vi "Grid_Monitor_V2backupblack.vi"(7 "Stop (In)":refnum<notifier>, 8 "Error (In)":errorcluster, 11 "SCADA AugState (In)":refnum<notifier>) -> (0 "Error (Out)":errorcluster, 3 "SCADA AugState (Out)":refnum<notifier>, 6 "Stop (Out)":refnum<notifier>)   [LabVIEW 2021]
uses:
  <vilib>/Utility/miscctls.llb/LVForegroundBackgroundColorsTypeDef.ctl
  SCADA/SCADA Augmented State.ctl
  Interval.ctl
  SCADA/SCADA Augmented State GUPTA.ctl
panel:
  out "V slider 11":T1(slide) caption="V-i" scale=230.0..240.0 scale format="%#_4g"
  out "V slider 25":dbl(slide) caption="V-i" max=-10.0 scale=720.0..750.0 scale format="%#_4g"
  out "V slider 24":dbl(slide) caption="V-i" max=-10.0 scale=720.0..750.0 scale format="%#_4g"
  out "V slider 23":dbl(slide) caption="V-i" max=-10.0 scale=720.0..750.0 scale format="%#_4g"
  out "V slider 22":dbl(slide) caption="V-i" max=-10.0 scale=720.0..750.0 scale format="%#_4g"
  out "V slider 21":dbl(slide) caption="V-i" max=-10.0 scale=720.0..750.0 scale format="%#_4g"
  out "V slider 20":dbl(slide) caption="V-i" max=-10.0 scale=720.0..750.0 scale format="%#_4g"
  out "V slider 19":dbl(slide) caption="V-i" max=-10.0 scale=720.0..750.0 scale format="%#_4g"
  out "V slider 18":dbl(slide) caption="V-i" max=-10.0 scale=720.0..750.0 scale format="%#_4g"
  out "V slider 17":T1(slide) caption="V-i" scale=230.0..240.0 scale format="%#_4g"
  out "V slider 16":T1(slide) caption="V-i" scale=230.0..240.0 scale format="%#_4g"
  out "V slider 15":T1(slide) caption="V-i" scale=230.0..240.0 scale format="%#_4g"
  out "V slider 14":T1(slide) caption="V-i" scale=230.0..240.0 scale format="%#_4g"
  out "V slider 13":T1(slide) caption="V-i" scale=230.0..240.0 scale format="%#_4g"
  out "V slider 12":T1(slide) caption="V-i" scale=230.0..240.0 scale format="%#_4g"
  out "V slider 10":T1(slide) caption="V-i" scale=230.0..240.0 scale format="%#_4g"
  out "V slider 9":T1(slide) caption="V-i" scale=230.0..240.0 scale format="%#_4g"
  out "V slider 8":T1(slide) caption="V-i" scale=230.0..240.0 scale format="%#_4g"
  out "V slider 7":T1(slide) caption="V-i" scale=230.0..240.0 scale format="%#_4g"
  out "V slider 6":T1(slide) caption="V-i" scale=230.0..240.0 scale format="%#_4g"
  out "V slider 4":T1(slide) caption="V-i" scale=230.0..240.0 scale format="%#_4g"
  out "V slider 3":T1(slide) caption="V-i" scale=230.0..240.0 scale format="%#_4g"
  out "V slider 1":T1(slide) caption="V-i" scale=230.0..240.0 scale format="%#_4g"
  out "V slider 0":T1(slide) caption="V-i" scale=230.0..240.0 scale format="%#_4g"
  out "size(s)":i32
  out "I slider 20":dbl(slide) min=-10.0 max=100.0 scale=0.0..100.0
  out "I slider 19":dbl(slide) min=-10.0 max=100.0 scale=0.0..100.0
  out "I slider 18":dbl(slide) min=-10.0 max=100.0 scale=0.0..100.0
  out "I slider 17":dbl(slide) min=-10.0 max=100.0 scale=0.0..100.0
  out "I slider 16":T1(slide) scale=0.0..44.0
  out "I slider 15":T1(slide) scale=0.0..44.0
  out "I slider 14":T1(slide) scale=0.0..44.0
  out "I slider 13":T1(slide) scale=0.0..44.0
  out "I slider 12":T1(slide) scale=0.0..108.0
  out "I slider 11":T1(slide) scale=0.0..82.0
  out "I slider 10":T1(slide) scale=0.0..82.0 scale format="%^#1.3g"
  out "I slider 9":T1(slide) scale=0.0..44.0
  out "I slider 8":T1(slide) scale=0.0..82.0 scale format="%^#1.3g"
  out "I slider 7":T1(slide) scale=0.0..207.0
  out "I slider 6":T1(slide) scale=0.0..135.0 scale format="%^#1.3g"
  out "I slider 5":T1(slide) scale=0.0..82.0
  out "I slider 4":T1(slide) scale=0.0..82.0
  out "I slider 3":T1(slide) scale=0.0..108.0
  out "I slider 2":T1(slide) scale=0.0..207.0 scale format="%^#1.3g"
  out "I slider 0":T1(slide) scale=0.0..207.0
  out "I slider 1":T1(slide) scale=0.0..44.0
  out "V slider 2":T1(slide) caption="V-i" scale=230.0..240.0 scale format="%#_4g"
  out "A":dbl caption="Numeric" format="%-^#10.3g"
  out "kW":dbl caption="Numeric" format="%#.3g"
  out "A":dbl caption="Numeric" format="%-^#10.3g"
  out "kW":dbl caption="Numeric" format="%#.3g"
  out "A":dbl caption="Numeric" format="%-^#10.3g"
  out "kW":dbl caption="Numeric" format="%#.3g"
  out "A":dbl caption="Numeric" format="%-^#10.3g"
  out "kW":dbl caption="Numeric" format="%#.3g"
  out "A":dbl caption="Numeric" format="%-^#10.3g"
  out "kW":dbl caption="Numeric" format="%#.3g"
  out "A":dbl caption="Numeric" format="%-^#10.3g"
  out "kW":dbl caption="Numeric" format="%#.3g"
  out "A":dbl caption="Numeric" format="%-^#10.3g"
  out "kW":dbl caption="Numeric" format="%#.3g"
  out "A":dbl caption="Numeric" format="%-^#10.3g"
  out "kW":dbl caption="Numeric" format="%#.3g"
  out "A":dbl[unit] caption="Numeric" format="%-^#10.3g"
  out "?VkVAr":dbl caption="Numeric" format="%.3g"
  out "kW":dbl caption="Numeric" format="%#.3g"
  out "A":dbl[unit] caption="Numeric" format="%-^#10.3g"
  out "?VkVAr":dbl caption="Numeric" format="%.3g"
  out "kW":dbl caption="Numeric" format="%#.3g"
  out "A":dbl[unit] caption="Numeric" format="%-^#10.3g"
  out "?VkVAr":dbl caption="Numeric" format="%.3g"
  out "kW":dbl caption="Numeric" format="%#.3g"
  out "A":dbl[unit] caption="Numeric" format="%-^#10.3g"
  out "?VkVAr":dbl caption="Numeric" format="%.3g"
  out "kW":dbl caption="Numeric" format="%#.3g"
  out "A":dbl[unit] caption="Numeric" format="%-^#10.3g"
  out "?VkVAr":dbl caption="Numeric" format="%.3g"
  out "kW":dbl caption="Numeric" format="%#.3g"
  out "A":dbl[unit] caption="Numeric" format="%-^#10.3g"
  out "?VkVAr":dbl caption="Numeric" format="%.3g"
  out "kW":dbl caption="Numeric" format="%#.3g"
  out "A":dbl[unit] caption="Numeric" format="%-^#10.3g"
  out "?VkVAr":dbl caption="Numeric" format="%.3g"
  out "kW":dbl caption="Numeric" format="%#.3g"
  out "A":dbl[unit] caption="Numeric" format="%-^#10.3g"
  out "?VkVAr":dbl caption="Numeric" format="%.3g"
  out "kW":dbl caption="Numeric" format="%#.3g"
  out "A":dbl[unit] caption="Numeric" format="%-^#10.3g"
  out "?VkVAr":dbl caption="Numeric" format="%.3g"
  out "kW":dbl caption="Numeric" format="%#.3g"
  out "A":dbl[unit] caption="Numeric" format="%-^#10.3g"
  out "?VkVAr":dbl caption="Numeric" format="%.3g"
  out "kW":dbl caption="Numeric" format="%#.3g"
  out "A2":dbl[unit] caption="Numeric" format="%-^#10.3g"
  out "?VkVAr":dbl caption="Numeric" format="%.3g"
  out "kW":dbl caption="Numeric" format="%#.3g"
  in  "Stop?":bool
  out "Connected?":bool
  out "AugState (Out)":refnum<notifier>
  in  "AugState (In)":refnum<notifier>
  # "B03"
  # "B01"
  # "B02"
  # "B05"
  # "B07"
  # "B14"
  # "B04"
  # "B06"
  # "B18"
  # "B22"
  # "B26"
  # "B08"
  # "B15"
  # "B19"
  # "B23"
  # "B09"
  # "B11"
  # "B10"
  # "B17"
  # "B21"
  # "B25"
  # "B13"
  # "B12"
  # "B16"
  # "B20"
  # "B24"
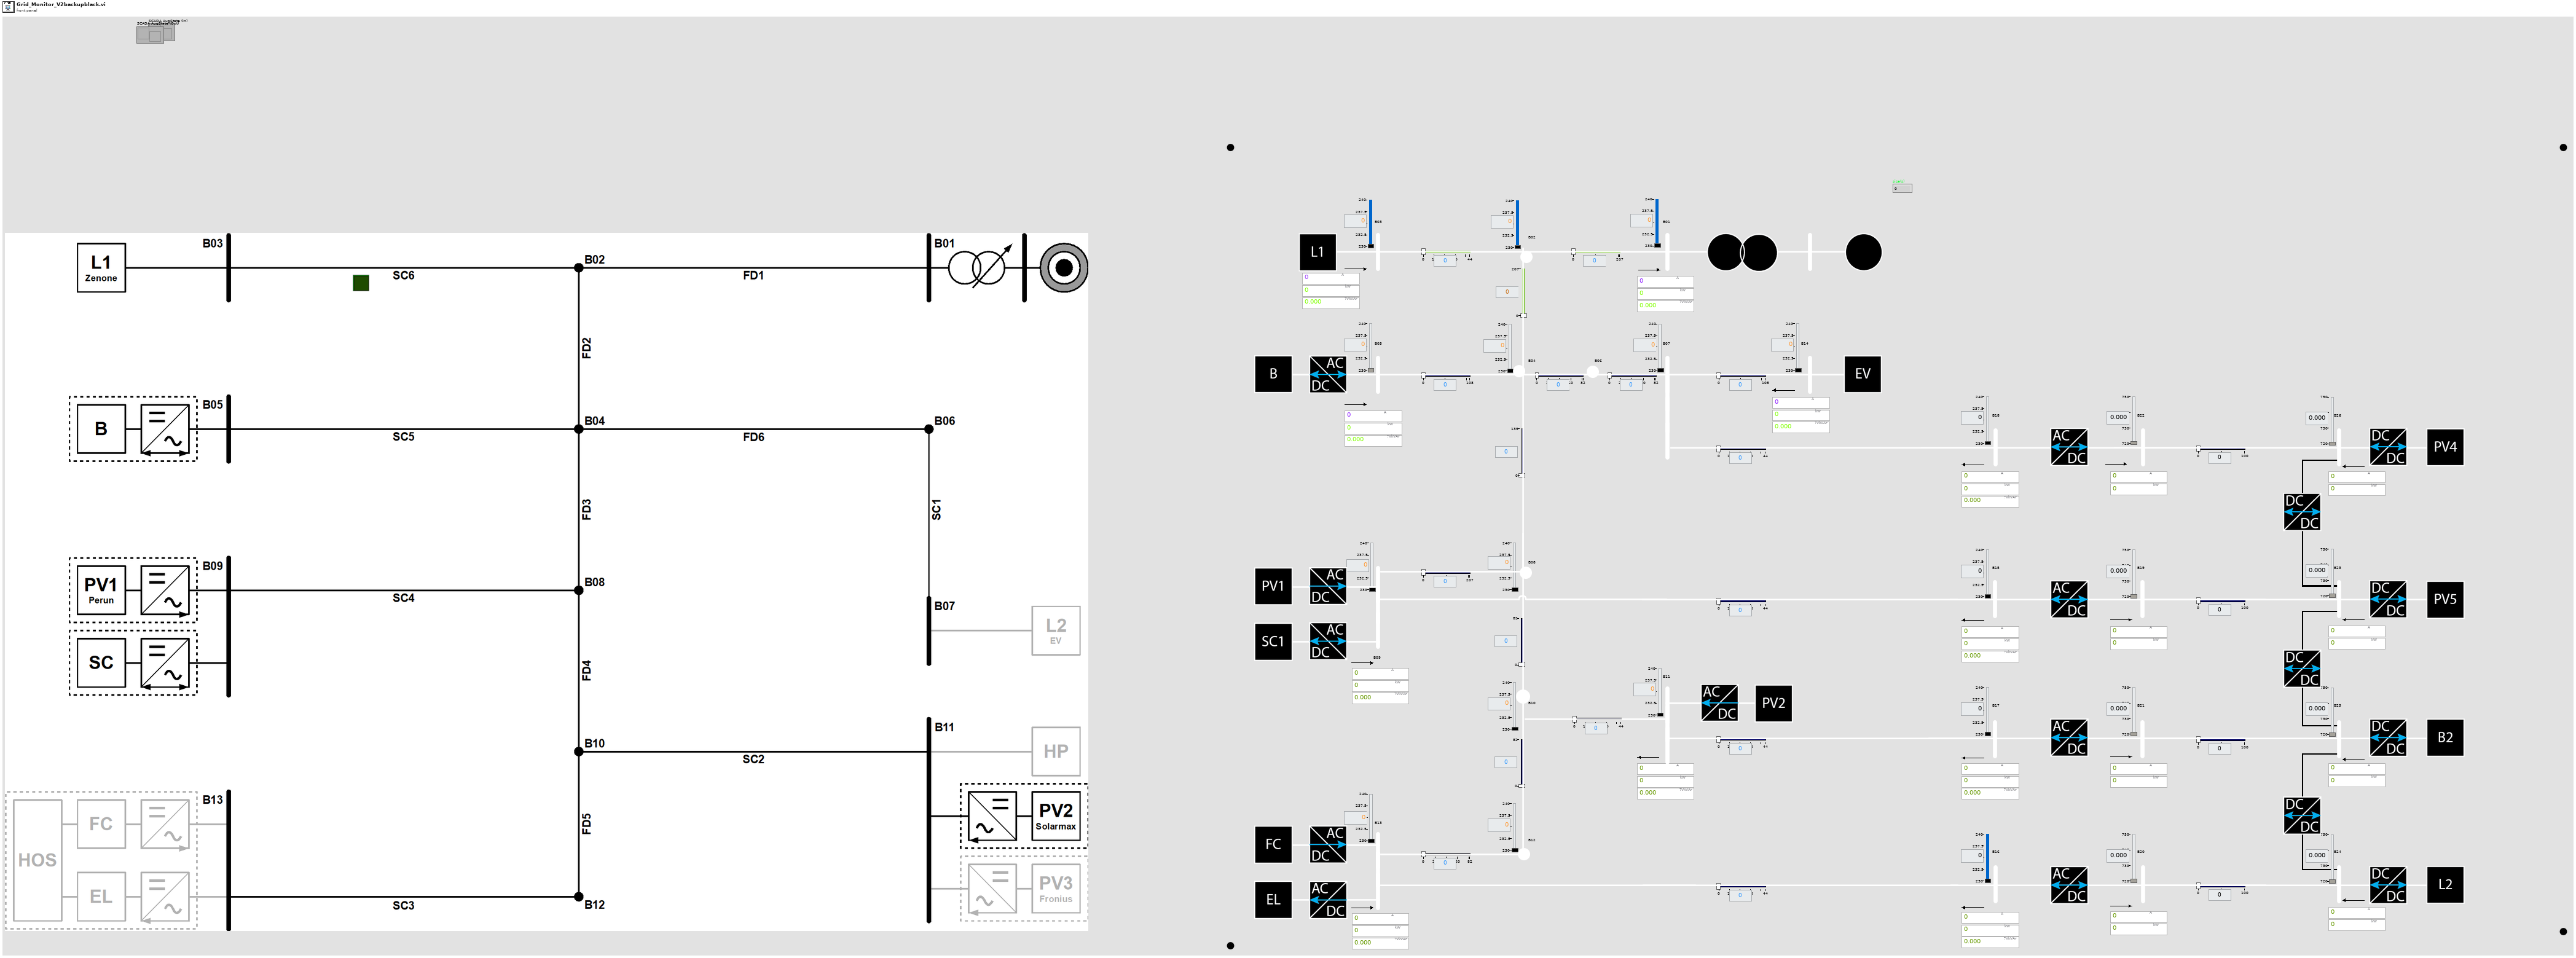
[diagram p1: front panel]
types:
  T1 = cluster{"Numeric":dbl, "Numeric":dbl, "Numeric":dbl}
  T2 = typedef "LVForegroundBackgroundColorsTypeDef.ctl" = cluster{"Foreground Color":u32, "Background Color":u32}
  T3 = typedef "SCADA Augmented State GUPTA.ctl" = cluster{"Buses":cluster{"Vbus":cdb[], "Iinjected":cdb[], "Sinjected":cdb[], "Vband":T4}[], "Lines":cluster{"Iforward":cdb[], "Ibackward":cdb[], "Imaximum":dbl}[], "f_downstream":dbl, "V_upstream":cdb[], "f_upstream":dbl, "Timestamp":timestamp, "M ":cluster{cdb, cdb, cdb}[], "z(k|k)":dbl[], "r(k)":dbl[]}
  T4 = typedef "Interval.ctl" = cluster{"lower":dbl, "upper":dbl}
  T5 = cluster{"Iforward":cdb[], "Ibackward":cdb[], "Imaximum":dbl}[]
  T6 = cluster{"Vbus":cdb[], "Iinjected":cdb[], "Sinjected":cdb[], "Vband":T4}[]
  T7 = cluster{"I_trip":dbl, "Phasor C":dbl, "Phasor C":dbl, "Phasor C":dbl}
  T8 = cluster{"V_maximum":dbl, "Phasor C":dbl, "Phasor C":dbl, "Phasor C":dbl, "V_minimun":dbl}
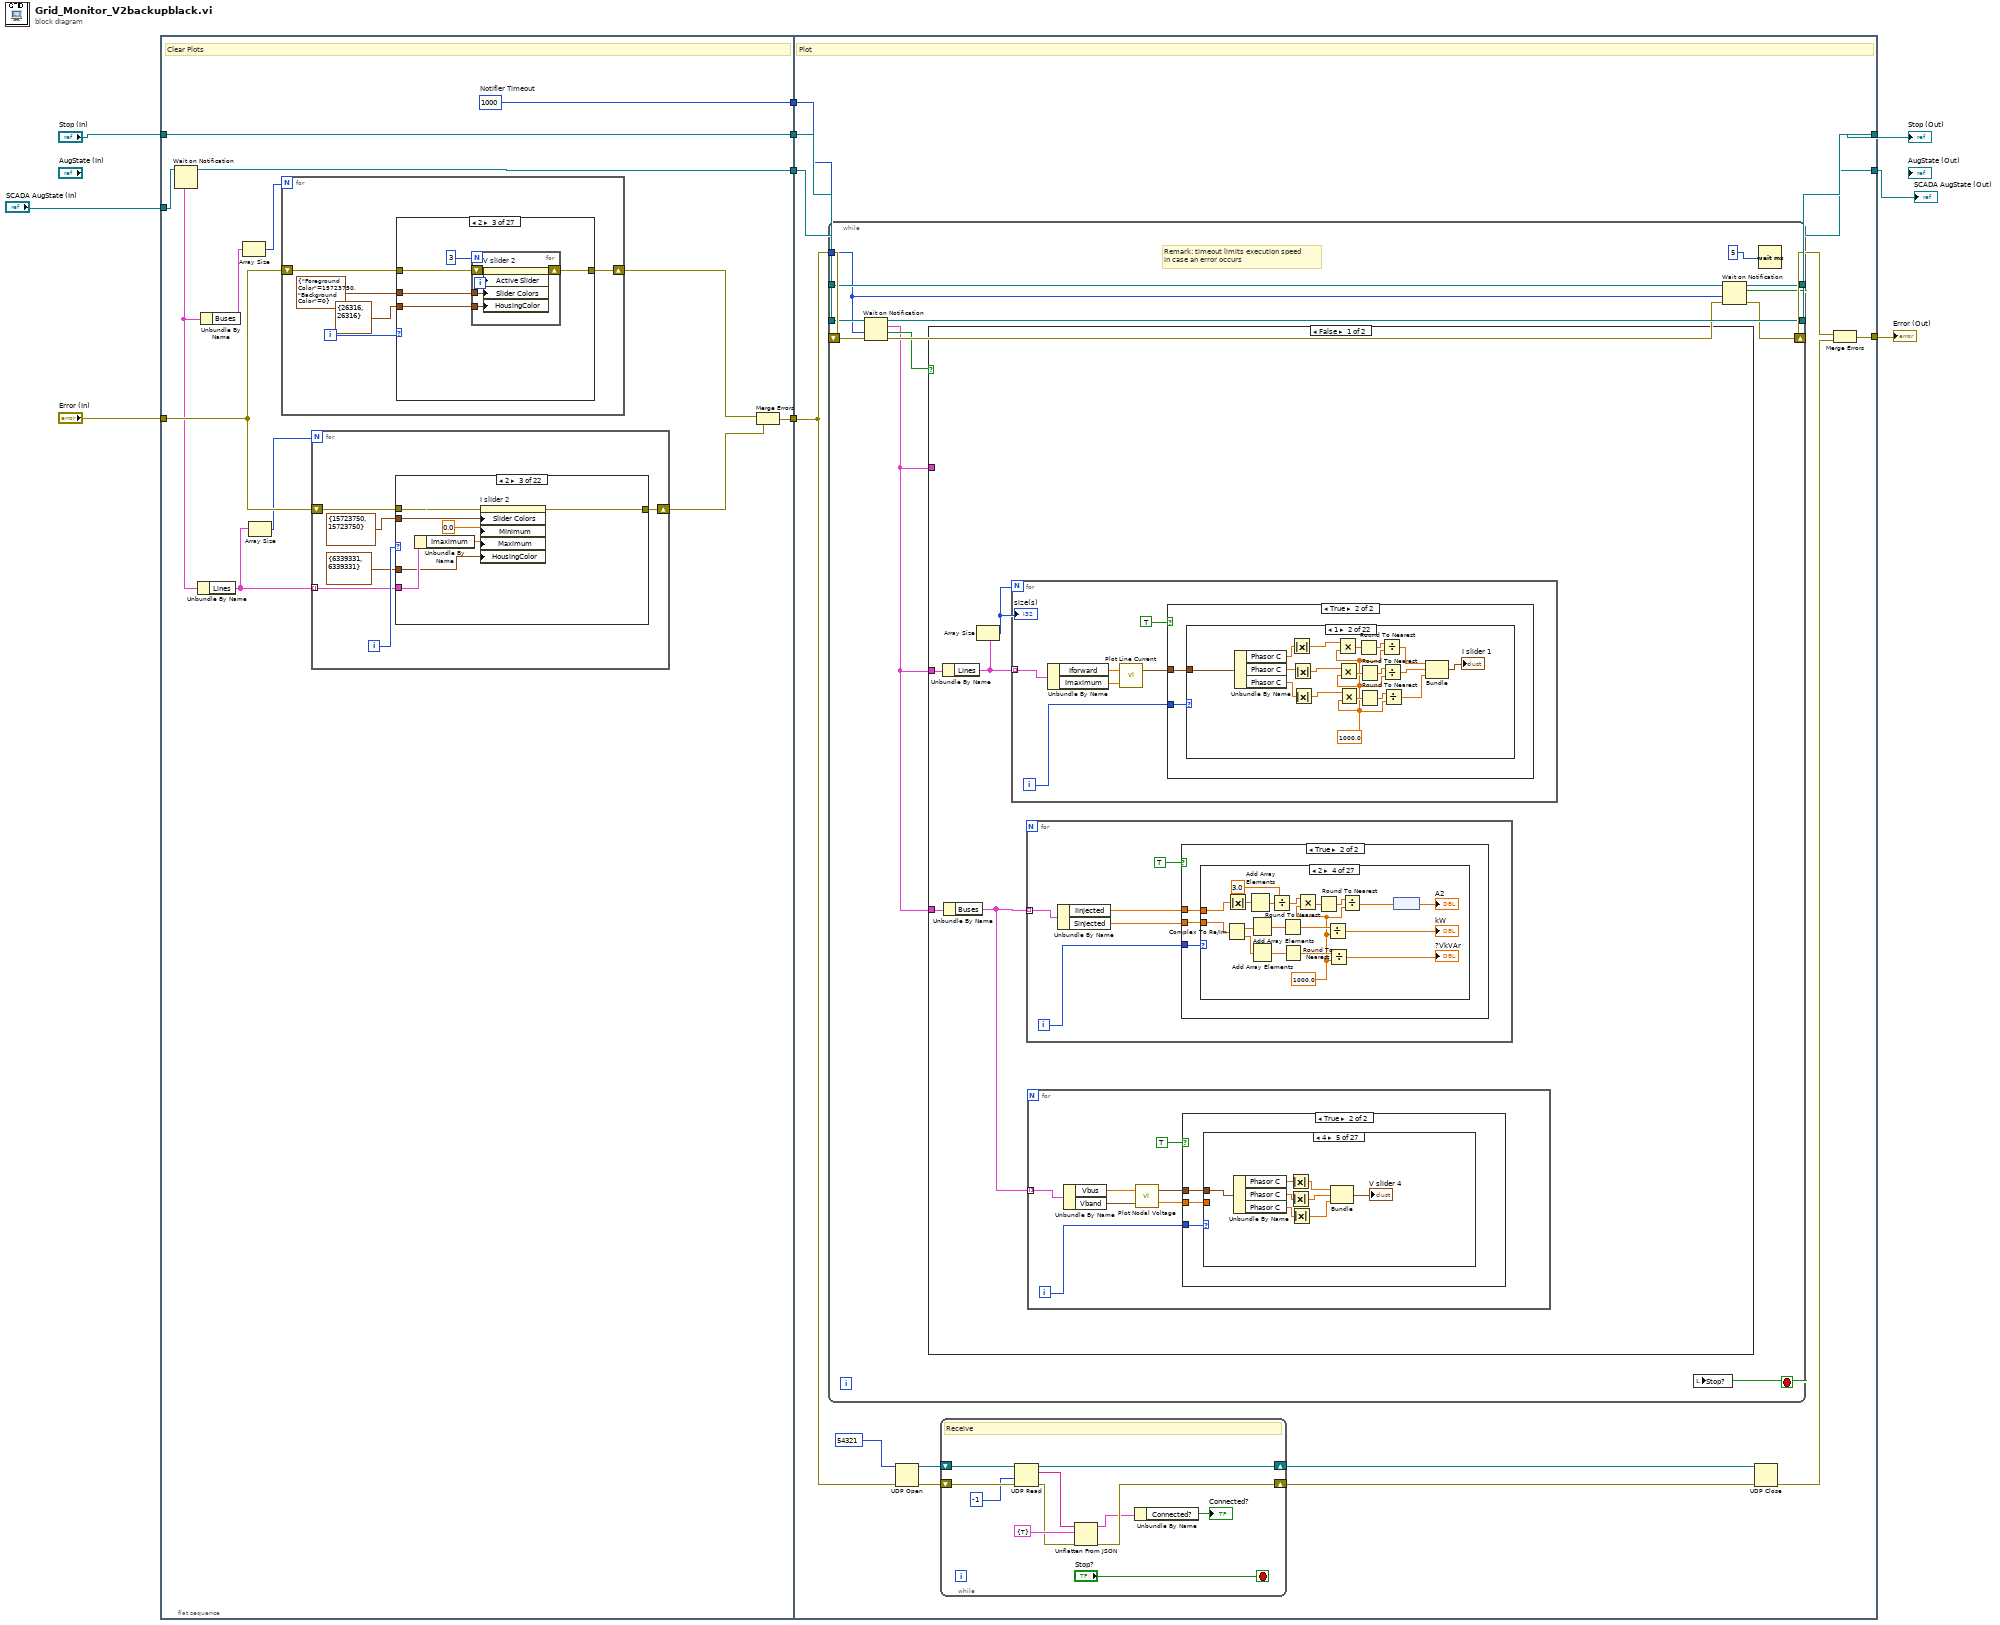
[diagram p0: block diagram]
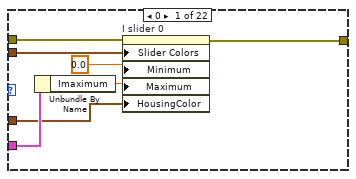
[diagram p2: hidden frame]
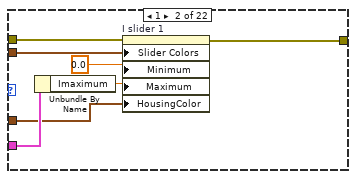
[diagram p3: hidden frame]
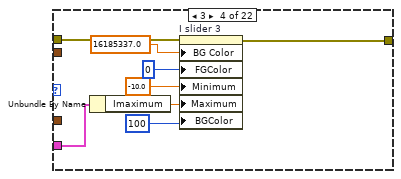
[diagram p4: hidden frame]
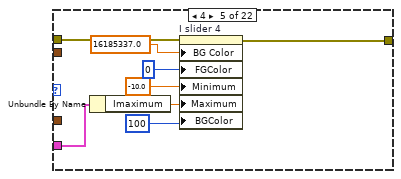
[diagram p5: hidden frame]
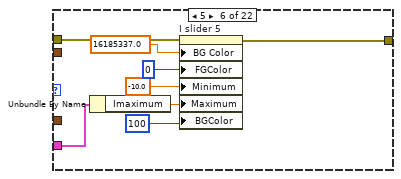
[diagram p6: hidden frame]
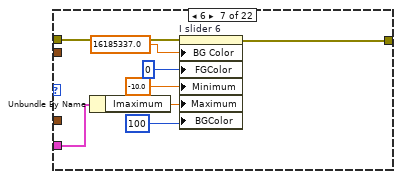
[diagram p7: hidden frame]
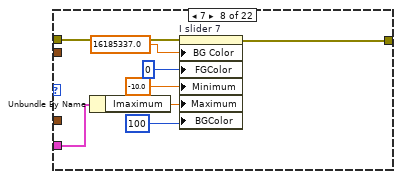
[diagram p8: hidden frame]
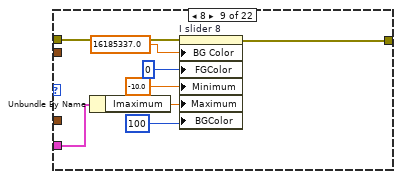
[diagram p9: hidden frame]
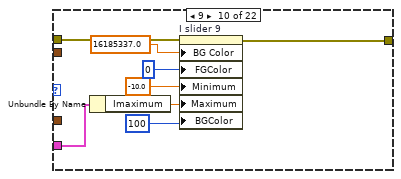
[diagram p10: hidden frame]
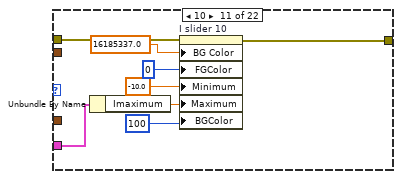
[diagram p11: hidden frame]
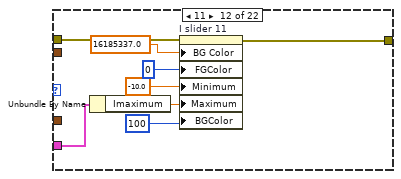
[diagram p12: hidden frame]
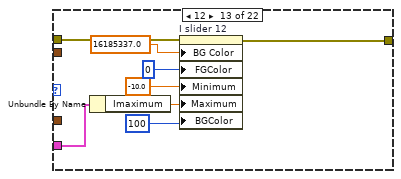
[diagram p13: hidden frame]
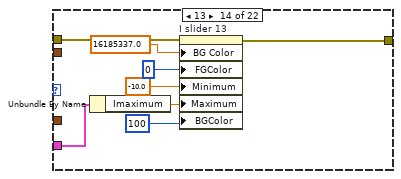
[diagram p14: hidden frame]
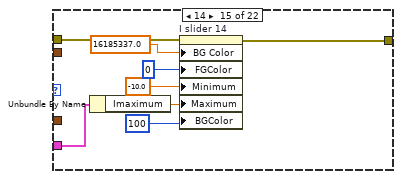
[diagram p15: hidden frame]
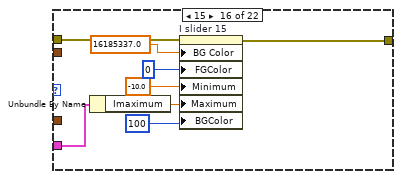
[diagram p16: hidden frame]
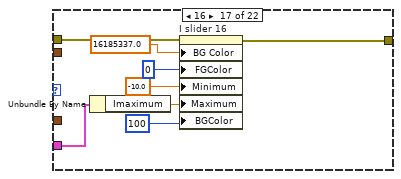
[diagram p17: hidden frame]
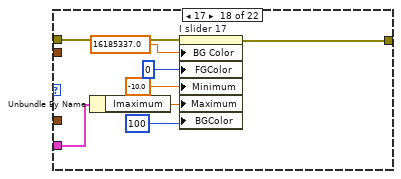
[diagram p18: hidden frame]
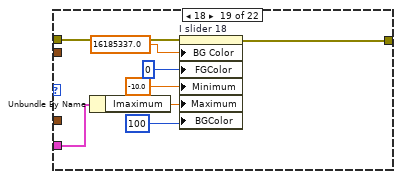
[diagram p19: hidden frame]
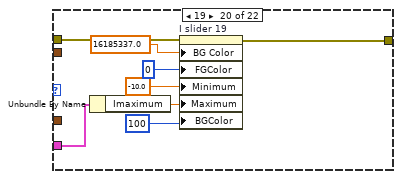
[diagram p20: hidden frame]
diagram:
  n1 = flat-sequence {
    tunnel: "Stop (In)" -> [w23]
    tunnel: [w16] -> w8
    tunnel: [w23] -> w7
    tunnel: [w20] -> w6
    tunnel: "Error (In)" -> [w19]
    tunnel: [w18] -> w3
    tunnel: "SCADA AugState (In)" -> [w17]
    tunnel: [w426] -> w9
    tunnel: [w417] -> w4
    tunnel: w8 -> [w428]
    tunnel: w7 -> [w427]
    tunnel: w6 -> [w419]
    tunnel: w3 -> [w425]
    tunnel: [w415] -> w2
    frame #0 {
      w18 = 1000  # Notifier Timeout
      # "Clear Plots"
      n2 = Wait on Notification(notifier=w17) -> (notifier out=w16:refnum<notifier>, notification=w13:T3)  [unwired: 3 in, 2 out]
      n3 = Unbundle By Name(w13) -> ("Lines"=w15:T5)
      n4 = Unbundle By Name(w13) -> ("Buses"=w12:T6)
      n5 = Array Size(array=w12) -> (size(s)=w11:i32)
      n6 = Array Size(array=w15) -> (size(s)=w14:i32)
      n7 = for {
        N: w11 -> [_]
        shift-right: [w198] -> w22
        shift-left: w19 -> [w200]
        i -> [w199]
        n8 = case shown="2" w199 {
          tunnel: w200 -> [w204 w214 w224 w233 w241 w249 w254 w262 w270 w278 w286 w294 w302 w310 w318 w327 w336 w344 w352 w360 w368 w376 w384 w392 w400 w408 w414]
          tunnel: [w205 w215 w225 w234 w242 w250 w255 w263 w271 w279 w287 w295 w303 w311 w319 w328 w337 w345 w353 w361 w369 w377 w385 w393 w401 w409 w414] -> w198
          tunnel: T2 {"Foreground Color"=15723750, "Background Color"=0} ("Slider Colors") -> [w202 w212 w222 w231 w239 w247 w252 w260 w268 w276 w284 w292 w300 w308 w316 w325 w334 w342 w350 w358 w366 w374 w382 w390 w398 w406 _]
          tunnel: T2 {"Foreground Color"=26316, "Background Color"=26316} ("Slider Colors") -> [w201 w211 w221 _ _ _ _ _ _ _ _ _ _ _ _ w324 _ _ _ _ _ _ _ _ _ _ _]
          frame 0 {
            n9 = for {
              N: 3 -> [_]
              tunnel: w202 -> [w208]
              shift-right: [w210] -> w205
              shift-left: w204 -> [w209]
              tunnel: w201 -> [w206]
              i -> [w207]
              n10 = property on="V slider 0" class="Slide (strict)"(error in=w209, "Active Slider"=w207, "Slider Colors"=w208, "HousingColor"=w206) -> (error out=w210:errorcluster)  [unwired: 1 in, 1 out]
            }
          }
          frame 1 {
            n11 = for {
              N: 3 -> [_]
              tunnel: w212 -> [w218]
              shift-right: [w220] -> w215
              shift-left: w214 -> [w219]
              tunnel: w211 -> [w216]
              i -> [w217]
              n12 = property on="V slider 1" class="Slide (strict)"(error in=w219, "Active Slider"=w217, "Slider Colors"=w218, "HousingColor"=w216) -> (error out=w220:errorcluster)  [unwired: 1 in, 1 out]
            }
          }
          frame 2 {
            n13 = for {
              N: 3 -> [_]
              tunnel: w222 -> [w228]
              shift-right: [w230] -> w225
              shift-left: w224 -> [w229]
              tunnel: w221 -> [w226]
              i -> [w227]
              n14 = property on="V slider 2" class="Slide (strict)"(error in=w229, "Active Slider"=w227, "Slider Colors"=w228, "HousingColor"=w226) -> (error out=w230:errorcluster)  [unwired: 1 in, 1 out]
            }
          }
          frame 3 {
            n15 = for {
              N: 3 -> [_]
              tunnel: w231 -> [w236]
              shift-right: [w238] -> w234
              shift-left: w233 -> [w237]
              i -> [w235]
              n16 = property on="V slider 3" class="Slide (strict)"(error in=w237, "Active Slider"=w235, "Slider Colors"=w236) -> (error out=w238:errorcluster)  [unwired: 1 in, 1 out]
            }
          }
          frame 4 {
            n17 = for {
              N: 3 -> [_]
              tunnel: w239 -> [w244]
              shift-right: [w246] -> w242
              shift-left: w241 -> [w245]
              i -> [w243]
              n18 = property on="I slider 4" class="Slide (strict)"(error in=w245, "Active Slider"=w243, "Slider Colors"=w244) -> (error out=w246:errorcluster)  [unwired: 1 in, 1 out]
            }
          }
          frame 5 {
            n19 = for {
              N: 3 -> [_]
              tunnel: w247 -> [_]
              shift-right: [w251] -> w250
              shift-left: w249 -> [w251]
            }
          }
          frame 6 {
            n20 = for {
              N: 3 -> [_]
              tunnel: w252 -> [w257]
              shift-right: [w259] -> w255
              shift-left: w254 -> [w258]
              i -> [w256]
              n21 = property on="V slider 6" class="Slide (strict)"(error in=w258, "Active Slider"=w256, "Slider Colors"=w257) -> (error out=w259:errorcluster)  [unwired: 1 in, 1 out]
            }
          }
          frame 7 {
            n22 = for {
              N: 3 -> [_]
              tunnel: w260 -> [w265]
              shift-right: [w267] -> w263
              shift-left: w262 -> [w266]
              i -> [w264]
              n23 = property on="V slider 7" class="Slide (strict)"(error in=w266, "Active Slider"=w264, "Slider Colors"=w265) -> (error out=w267:errorcluster)  [unwired: 1 in, 1 out]
            }
          }
          frame 8 {
            n24 = for {
              N: 3 -> [_]
              tunnel: w268 -> [w273]
              shift-right: [w275] -> w271
              shift-left: w270 -> [w274]
              i -> [w272]
              n25 = property on="V slider 8" class="Slide (strict)"(error in=w274, "Active Slider"=w272, "Slider Colors"=w273) -> (error out=w275:errorcluster)  [unwired: 1 in, 1 out]
            }
          }
          frame 9 {
            n26 = for {
              N: 3 -> [_]
              tunnel: w276 -> [w281]
              shift-right: [w283] -> w279
              shift-left: w278 -> [w282]
              i -> [w280]
              n27 = property on="V slider 9" class="Slide (strict)"(error in=w282, "Active Slider"=w280, "Slider Colors"=w281) -> (error out=w283:errorcluster)  [unwired: 1 in, 1 out]
            }
          }
          frame 10 {
            n28 = for {
              N: 3 -> [_]
              tunnel: w284 -> [w289]
              shift-right: [w291] -> w287
              shift-left: w286 -> [w290]
              i -> [w288]
              n29 = property on="V slider 10" class="Slide (strict)"(error in=w290, "Active Slider"=w288, "Slider Colors"=w289) -> (error out=w291:errorcluster)  [unwired: 1 in, 1 out]
            }
          }
          frame 11 {
            n30 = for {
              N: 3 -> [_]
              tunnel: w292 -> [w296]
              shift-right: [w298] -> w295
              shift-left: w294 -> [w299]
              i -> [w297]
              n31 = property on="V slider 11" class="Slide (strict)"(error in=w299, "Active Slider"=w297, "Slider Colors"=w296) -> (error out=w298:errorcluster)  [unwired: 1 in, 1 out]
            }
          }
          frame 12 {
            n32 = for {
              N: 3 -> [_]
              tunnel: w300 -> [w305]
              shift-right: [w307] -> w303
              shift-left: w302 -> [w306]
              i -> [w304]
              n33 = property on="V slider 12" class="Slide (strict)"(error in=w306, "Active Slider"=w304, "Slider Colors"=w305) -> (error out=w307:errorcluster)  [unwired: 1 in, 1 out]
            }
          }
          frame 13 {
            n34 = for {
              N: 3 -> [_]
              tunnel: w308 -> [w313]
              shift-right: [w315] -> w311
              shift-left: w310 -> [w314]
              i -> [w312]
              n35 = property on="V slider 13" class="Slide (strict)"(error in=w314, "Active Slider"=w312, "Slider Colors"=w313) -> (error out=w315:errorcluster)  [unwired: 1 in, 1 out]
            }
          }
          frame 14 {
            n36 = for {
              N: 3 -> [_]
              tunnel: w316 -> [w321]
              shift-right: [w323] -> w319
              shift-left: w318 -> [w322]
              i -> [w320]
              n37 = property on="V slider 14" class="Slide (strict)"(error in=w322, "Active Slider"=w320, "Slider Colors"=w321) -> (error out=w323:errorcluster)  [unwired: 1 in, 1 out]
            }
          }
          frame 15 {
            n38 = for {
              N: 3 -> [_]
              tunnel: w325 -> [w331]
              shift-right: [w333] -> w328
              shift-left: w327 -> [w332]
              tunnel: w324 -> [w329]
              i -> [w330]
              n39 = property on="V slider 15" class="Slide (strict)"(error in=w332, "Active Slider"=w330, "Slider Colors"=w331, "HousingColor"=w329) -> (error out=w333:errorcluster)  [unwired: 1 in, 1 out]
            }
          }
          frame 16 {
            n40 = for {
              N: 3 -> [_]
              tunnel: w334 -> [w339]
              shift-right: [w341] -> w337
              shift-left: w336 -> [w340]
              i -> [w338]
              n41 = property on="V slider 16" class="Slide (strict)"(error in=w340, "Active Slider"=w338, "Slider Colors"=w339) -> (error out=w341:errorcluster)  [unwired: 1 in, 1 out]
            }
          }
          frame 17 {
            n42 = for {
              N: 3 -> [_]
              tunnel: w342 -> [w347]
              shift-right: [w349] -> w345
              shift-left: w344 -> [w348]
              i -> [w346]
              n43 = property on="V slider 17" class="Slide (strict)"(error in=w348, "Active Slider"=w346, "Slider Colors"=w347) -> (error out=w349:errorcluster)  [unwired: 1 in, 1 out]
            }
          }
          frame 18 {
            n44 = for {
              N: 1 -> [_]
              shift-right: [w357] -> w353
              shift-left: w352 -> [w356]
              tunnel: w350 -> [w354]
              i -> [w355]
              n45 = property on="V slider 18" class="Slide (strict)"(error in=w356, "Active Slider"=w355, "Slider Colors"=w354) -> (error out=w357:errorcluster)  [unwired: 1 in, 1 out]
            }
          }
          frame 19 {
            n46 = for {
              N: 1 -> [_]
              tunnel: w358 -> [w363]
              shift-right: [w365] -> w361
              shift-left: w360 -> [w364]
              i -> [w362]
              n47 = property on="V slider 19" class="Slide (strict)"(error in=w364, "Active Slider"=w362, "Slider Colors"=w363) -> (error out=w365:errorcluster)  [unwired: 1 in, 1 out]
            }
          }
          frame 20 {
            n48 = for {
              N: 1 -> [_]
              tunnel: w366 -> [w371]
              shift-right: [w373] -> w369
              shift-left: w368 -> [w372]
              i -> [w370]
              n49 = property on="V slider 20" class="Slide (strict)"(error in=w372, "Active Slider"=w370, "Slider Colors"=w371) -> (error out=w373:errorcluster)  [unwired: 1 in, 1 out]
            }
          }
          frame 21 {
            n50 = for {
              N: 1 -> [_]
              tunnel: w374 -> [w379]
              shift-right: [w381] -> w377
              shift-left: w376 -> [w380]
              i -> [w378]
              n51 = property on="V slider 21" class="Slide (strict)"(error in=w380, "Active Slider"=w378, "Slider Colors"=w379) -> (error out=w381:errorcluster)  [unwired: 1 in, 1 out]
            }
          }
          frame 22 {
            n52 = for {
              N: 1 -> [_]
              tunnel: w382 -> [w387]
              shift-right: [w389] -> w385
              shift-left: w384 -> [w388]
              i -> [w386]
              n53 = property on="V slider 22" class="Slide (strict)"(error in=w388, "Active Slider"=w386, "Slider Colors"=w387) -> (error out=w389:errorcluster)  [unwired: 1 in, 1 out]
            }
          }
          frame 23 {
            n54 = for {
              N: 1 -> [_]
              tunnel: w390 -> [w395]
              shift-right: [w397] -> w393
              shift-left: w392 -> [w396]
              i -> [w394]
              n55 = property on="V slider 23" class="Slide (strict)"(error in=w396, "Active Slider"=w394, "Slider Colors"=w395) -> (error out=w397:errorcluster)  [unwired: 1 in, 1 out]
            }
          }
          frame 24 {
            n56 = for {
              N: 1 -> [_]
              tunnel: w398 -> [w403]
              shift-right: [w405] -> w401
              shift-left: w400 -> [w404]
              i -> [w402]
              n57 = property on="V slider 24" class="Slide (strict)"(error in=w404, "Active Slider"=w402, "Slider Colors"=w403) -> (error out=w405:errorcluster)  [unwired: 1 in, 1 out]
            }
          }
          frame 25 {
            n58 = for {
              N: 1 -> [_]
              tunnel: w406 -> [w411]
              shift-right: [w413] -> w409
              shift-left: w408 -> [w412]
              i -> [w410]
              n59 = property on="V slider 25" class="Slide (strict)"(error in=w412, "Active Slider"=w410, "Slider Colors"=w411) -> (error out=w413:errorcluster)  [unwired: 1 in, 1 out]
            }
          }
          frame 26, Default {
          }
        }
      }
      n60 = for {
        N: w14 -> [_]
        shift-right: [w27] -> w21
        shift-left: w19 -> [w29]
        tunnel: w15 -> [w26] mode=indexing
        i -> [w28]
        n61 = case shown="2" w28 {
          tunnel: w29 -> [w36 w43 w50 w57 w65 w73 w81 w89 w97 w105 w113 w121 w129 w137 w145 w153 w161 w169 w177 w185 w193 w195]
          tunnel: [w33 w40 w47 w51 w59 w67 w75 w83 w91 w99 w107 w115 w123 w131 w139 w147 w155 w163 w171 w179 w187 w195] -> w27
          tunnel: w26 -> [w34 w41 w48 w53 w61 w69 w77 w85 w93 w101 w109 w117 w125 w133 w141 w149 w157 w165 w173 w181 w189 _]
          tunnel: T2 {"Foreground Color"=6339331, "Background Color"=6339331} ("Slider Colors") -> [w31 w38 w45 _ _ _ _ _ _ _ _ _ _ _ _ _ _ _ _ _ _ _]
          tunnel: T2 {"Foreground Color"=15723750, "Background Color"=15723750} ("Slider Colors") -> [w30 w37 w44 _ _ _ _ _ _ _ _ _ _ _ _ _ _ _ _ _ _ _]
          frame 0 {
            n62 = Unbundle By Name(w34) -> ("Imaximum"=w32:dbl)
            n63 = property on="I slider 0" class="Slide (strict)"(error in=w36, "Slider Colors"=w30, "Minimum"=0.0 ("Data Entry Limits:Minimum"), "Maximum"=w32, "HousingColor"=w31) -> (error out=w33:errorcluster)  [unwired: 1 in, 1 out]
          }
          frame 1 {
            n64 = Unbundle By Name(w41) -> ("Imaximum"=w39:dbl)
            n65 = property on="I slider 1" class="Slide (strict)"(error in=w43, "Slider Colors"=w37, "Minimum"=0.0 ("Data Entry Limits:Minimum"), "Maximum"=w39, "HousingColor"=w38) -> (error out=w40:errorcluster)  [unwired: 1 in, 1 out]
          }
          frame 2 {
            n66 = Unbundle By Name(w48) -> ("Imaximum"=w46:dbl)
            n67 = property on="I slider 2" class="Slide (strict)"(error in=w50, "Slider Colors"=w44, "Minimum"=0.0 ("Data Entry Limits:Minimum"), "Maximum"=w46, "HousingColor"=w45) -> (error out=w47:errorcluster)  [unwired: 1 in, 1 out]
          }
          frame 3 {
            n68 = Unbundle By Name(w53) -> ("Imaximum"=w52:dbl)
            n69 = property on="I slider 3" class="Slide (strict)"(error in=w57, "BG Color"=16185337.0 ("Plot Area:Colors:BG Color"), "FGColor"=u32 0 ("Plot Area:Colors:FG Color"), "Minimum"=-10.0 ("Data Entry Limits:Minimum"), "Maximum"=w52, "BGColor"=u32 100 ("Housing Colors:BG Color")) -> (error out=w51:errorcluster)  [unwired: 1 in, 1 out]
          }
          frame 4 {
            n70 = Unbundle By Name(w61) -> ("Imaximum"=w60:dbl)
            n71 = property on="I slider 4" class="Slide (strict)"(error in=w65, "BG Color"=16185337.0 ("Plot Area:Colors:BG Color"), "FGColor"=u32 0 ("Plot Area:Colors:FG Color"), "Minimum"=-10.0 ("Data Entry Limits:Minimum"), "Maximum"=w60, "BGColor"=u32 100 ("Housing Colors:BG Color")) -> (error out=w59:errorcluster)  [unwired: 1 in, 1 out]
          }
          frame 5 {
            n72 = Unbundle By Name(w69) -> ("Imaximum"=w68:dbl)
            n73 = property on="I slider 5" class="Slide (strict)"(error in=w73, "BG Color"=16185337.0 ("Plot Area:Colors:BG Color"), "FGColor"=u32 0 ("Plot Area:Colors:FG Color"), "Minimum"=-10.0 ("Data Entry Limits:Minimum"), "Maximum"=w68, "BGColor"=u32 100 ("Housing Colors:BG Color")) -> (error out=w67:errorcluster)  [unwired: 1 in, 1 out]
          }
          frame 6 {
            n74 = Unbundle By Name(w77) -> ("Imaximum"=w76:dbl)
            n75 = property on="I slider 6" class="Slide (strict)"(error in=w81, "BG Color"=16185337.0 ("Plot Area:Colors:BG Color"), "FGColor"=u32 0 ("Plot Area:Colors:FG Color"), "Minimum"=-10.0 ("Data Entry Limits:Minimum"), "Maximum"=w76, "BGColor"=u32 100 ("Housing Colors:BG Color")) -> (error out=w75:errorcluster)  [unwired: 1 in, 1 out]
          }
          frame 7 {
            n76 = Unbundle By Name(w85) -> ("Imaximum"=w84:dbl)
            n77 = property on="I slider 7" class="Slide (strict)"(error in=w89, "BG Color"=16185337.0 ("Plot Area:Colors:BG Color"), "FGColor"=u32 0 ("Plot Area:Colors:FG Color"), "Minimum"=-10.0 ("Data Entry Limits:Minimum"), "Maximum"=w84, "BGColor"=u32 100 ("Housing Colors:BG Color")) -> (error out=w83:errorcluster)  [unwired: 1 in, 1 out]
          }
          frame 8 {
            n78 = Unbundle By Name(w93) -> ("Imaximum"=w92:dbl)
            n79 = property on="I slider 8" class="Slide (strict)"(error in=w97, "BG Color"=16185337.0 ("Plot Area:Colors:BG Color"), "FGColor"=u32 0 ("Plot Area:Colors:FG Color"), "Minimum"=-10.0 ("Data Entry Limits:Minimum"), "Maximum"=w92, "BGColor"=u32 100 ("Housing Colors:BG Color")) -> (error out=w91:errorcluster)  [unwired: 1 in, 1 out]
          }
          frame 9 {
            n80 = Unbundle By Name(w101) -> ("Imaximum"=w100:dbl)
            n81 = property on="I slider 9" class="Slide (strict)"(error in=w105, "BG Color"=16185337.0 ("Plot Area:Colors:BG Color"), "FGColor"=u32 0 ("Plot Area:Colors:FG Color"), "Minimum"=-10.0 ("Data Entry Limits:Minimum"), "Maximum"=w100, "BGColor"=u32 100 ("Housing Colors:BG Color")) -> (error out=w99:errorcluster)  [unwired: 1 in, 1 out]
          }
          frame 10 {
            n82 = Unbundle By Name(w109) -> ("Imaximum"=w108:dbl)
            n83 = property on="I slider 10" class="Slide (strict)"(error in=w113, "BG Color"=16185337.0 ("Plot Area:Colors:BG Color"), "FGColor"=u32 0 ("Plot Area:Colors:FG Color"), "Minimum"=-10.0 ("Data Entry Limits:Minimum"), "Maximum"=w108, "BGColor"=u32 100 ("Housing Colors:BG Color")) -> (error out=w107:errorcluster)  [unwired: 1 in, 1 out]
          }
          frame 11 {
            n84 = Unbundle By Name(w117) -> ("Imaximum"=w116:dbl)
            n85 = property on="I slider 11" class="Slide (strict)"(error in=w121, "BG Color"=16185337.0 ("Plot Area:Colors:BG Color"), "FGColor"=u32 0 ("Plot Area:Colors:FG Color"), "Minimum"=-10.0 ("Data Entry Limits:Minimum"), "Maximum"=w116, "BGColor"=u32 100 ("Housing Colors:BG Color")) -> (error out=w115:errorcluster)  [unwired: 1 in, 1 out]
          }
          frame 12 {
            n86 = Unbundle By Name(w125) -> ("Imaximum"=w124:dbl)
            n87 = property on="I slider 12" class="Slide (strict)"(error in=w129, "BG Color"=16185337.0 ("Plot Area:Colors:BG Color"), "FGColor"=u32 0 ("Plot Area:Colors:FG Color"), "Minimum"=-10.0 ("Data Entry Limits:Minimum"), "Maximum"=w124, "BGColor"=u32 100 ("Housing Colors:BG Color")) -> (error out=w123:errorcluster)  [unwired: 1 in, 1 out]
          }
          frame 13 {
            n88 = Unbundle By Name(w133) -> ("Imaximum"=w132:dbl)
            n89 = property on="I slider 13" class="Slide (strict)"(error in=w137, "BG Color"=16185337.0 ("Plot Area:Colors:BG Color"), "FGColor"=u32 0 ("Plot Area:Colors:FG Color"), "Minimum"=-10.0 ("Data Entry Limits:Minimum"), "Maximum"=w132, "BGColor"=u32 100 ("Housing Colors:BG Color")) -> (error out=w131:errorcluster)  [unwired: 1 in, 1 out]
          }
          frame 14 {
            n90 = Unbundle By Name(w141) -> ("Imaximum"=w140:dbl)
            n91 = property on="I slider 14" class="Slide (strict)"(error in=w145, "BG Color"=16185337.0 ("Plot Area:Colors:BG Color"), "FGColor"=u32 0 ("Plot Area:Colors:FG Color"), "Minimum"=-10.0 ("Data Entry Limits:Minimum"), "Maximum"=w140, "BGColor"=u32 100 ("Housing Colors:BG Color")) -> (error out=w139:errorcluster)  [unwired: 1 in, 1 out]
          }
          frame 15 {
            n92 = Unbundle By Name(w149) -> ("Imaximum"=w148:dbl)
            n93 = property on="I slider 15" class="Slide (strict)"(error in=w153, "BG Color"=16185337.0 ("Plot Area:Colors:BG Color"), "FGColor"=u32 0 ("Plot Area:Colors:FG Color"), "Minimum"=-10.0 ("Data Entry Limits:Minimum"), "Maximum"=w148, "BGColor"=u32 100 ("Housing Colors:BG Color")) -> (error out=w147:errorcluster)  [unwired: 1 in, 1 out]
          }
          frame 16 {
            n94 = Unbundle By Name(w157) -> ("Imaximum"=w156:dbl)
            n95 = property on="I slider 16" class="Slide (strict)"(error in=w161, "BG Color"=16185337.0 ("Plot Area:Colors:BG Color"), "FGColor"=u32 0 ("Plot Area:Colors:FG Color"), "Minimum"=-10.0 ("Data Entry Limits:Minimum"), "Maximum"=w156, "BGColor"=u32 100 ("Housing Colors:BG Color")) -> (error out=w155:errorcluster)  [unwired: 1 in, 1 out]
          }
          frame 17 {
            n96 = Unbundle By Name(w165) -> ("Imaximum"=w164:dbl)
            n97 = property on="I slider 17" class="Slide (strict)"(error in=w169, "BG Color"=16185337.0 ("Plot Area:Colors:BG Color"), "FGColor"=u32 0 ("Plot Area:Colors:FG Color"), "Minimum"=-10.0 ("Data Entry Limits:Minimum"), "Maximum"=w164, "BGColor"=u32 100 ("Housing Colors:BG Color")) -> (error out=w163:errorcluster)  [unwired: 1 in, 1 out]
          }
          frame 18 {
            n98 = Unbundle By Name(w173) -> ("Imaximum"=w172:dbl)
            n99 = property on="I slider 18" class="Slide (strict)"(error in=w177, "BG Color"=16185337.0 ("Plot Area:Colors:BG Color"), "FGColor"=u32 0 ("Plot Area:Colors:FG Color"), "Minimum"=-10.0 ("Data Entry Limits:Minimum"), "Maximum"=w172, "BGColor"=u32 100 ("Housing Colors:BG Color")) -> (error out=w171:errorcluster)  [unwired: 1 in, 1 out]
          }
          frame 19 {
            n100 = Unbundle By Name(w181) -> ("Imaximum"=w180:dbl)
            n101 = property on="I slider 19" class="Slide (strict)"(error in=w185, "BG Color"=16185337.0 ("Plot Area:Colors:BG Color"), "FGColor"=u32 0 ("Plot Area:Colors:FG Color"), "Minimum"=-10.0 ("Data Entry Limits:Minimum"), "Maximum"=w180, "BGColor"=u32 100 ("Housing Colors:BG Color")) -> (error out=w179:errorcluster)  [unwired: 1 in, 1 out]
          }
          frame 20 {
            n102 = Unbundle By Name(w189) -> ("Imaximum"=w188:dbl)
            n103 = property on="I slider 20" class="Slide (strict)"(error in=w193, "BG Color"=16185337.0 ("Plot Area:Colors:BG Color"), "FGColor"=u32 0 ("Plot Area:Colors:FG Color"), "Minimum"=-10.0 ("Data Entry Limits:Minimum"), "Maximum"=w188, "BGColor"=u32 100 ("Housing Colors:BG Color")) -> (error out=w187:errorcluster)  [unwired: 1 in, 1 out]
          }
          frame 21, Default {
          }
        }
      }
      n104 = Merge Errors(w22, w21) -> (w20:errorcluster)
    }
    frame #1 {
      # "Plot"
      n105 = while {
        tunnel: w428 -> [w451]
        shift-right: [w445] -> w418
        shift-left: w419 -> [w450]
        tunnel: [w449] -> w415
        tunnel: w427 -> [w448]
        tunnel: [w447] -> w426
        tunnel: w425 -> [w442]
        stop <- w441 stop-if-true
        # "Remark: timeout limits execution speed\nin case an error occurs"
        n106 = Wait on Notification(notifier=w451, timeout in ms (-1)=w442, error in (no error)=w450) -> (notifier out=w449:refnum<notifier>, notification=w440:T3, timed out?=w444:bool, error out=w446:errorcluster)  [unwired: 1 in]
        n107 = case shown="False" w444 {
          tunnel: w440 -> [_ _]
          tunnel: w440 -> [w456 _]
          tunnel: w440 -> [w455 _]
          frame False {
            n108 = Unbundle By Name(w456) -> ("Lines"=w453:T5)
            n109 = Unbundle By Name(w455) -> ("Buses"=w454:T6)
            n110 = Array Size(array=w453) -> (size(s)=w452:i32)
            "size(s)" <- w452
            n111 = for {
              N: w452 -> [_]
              tunnel: w453 -> [w1092] mode=indexing
              i -> [w1091]
              n112 = Unbundle By Name(w1092) -> ("Iforward"=w1089:cdb[], "Imaximum"=w1088:dbl)
              n113 = call "Plot Line Current.vi"("I_trip"=w1088, "I_line"=w1089) -> ("I-i"=w1090:T7)  [unwired: 1 in]
              n114 = case shown="True" TRUE {
                tunnel: w1091 -> [_ w1094]
                tunnel: w1090 -> [_ w1093]
                frame False {
                }
                frame True {
                  n115 = case shown="1" w1094 {
                    tunnel: w1093 -> [w1096 w1114 w1148 w1150 w1168 w1186 w1220 w1222 w1256 w1258 w1292 w1294 w1312 w1330 w1348 w1366 w1384 w1403 w1410 w1417 w1424 _]
                    frame 0 {
                      w1097 = 1000.0 ("y")
                      n116 = Unbundle By Name(w1096) -> ("Phasor C"=w1109:dbl, "Phasor C"=w1103:dbl, "Phasor C"=w1101:dbl)
                      n117 = Absolute Value(x=w1109) -> (abs(x)=w1110:dbl)
                      n118 = Absolute Value(x=w1103) -> (abs(x)=w1102:dbl)
                      n119 = Absolute Value(x=w1101) -> (abs(x)=w1100:dbl)
                      n120 = Multiply(x=w1110, y=w1097) -> (x*y=w1111:dbl)
                      n121 = Multiply(x=w1102, y=w1097) -> (x*y=w1106:dbl)
                      n122 = Multiply(x=w1100, y=w1097) -> (x*y=w1104:dbl)
                      n123 = Round To Nearest(number=w1111) -> (nearest integer value=w1112:dbl)
                      n124 = Round To Nearest(number=w1106) -> (nearest integer value=w1107:dbl)
                      n125 = Round To Nearest(number=w1104) -> (nearest integer value=w1105:dbl)
                      n126 = Divide(x=w1112, y=w1097) -> (x/y=w1108:dbl)
                      n127 = Divide(x=w1107, y=w1097) -> (x/y=w1099:dbl)
                      n128 = Divide(x=w1105, y=w1097) -> (x/y=w1098:dbl)
                      n129 = Bundle(w1108, w1099, w1098) -> (→"I slider 0":cluster{dbl, dbl, dbl})  [unwired: 1 in]
                    }
                    frame 1 {
                      w1115 = 1000.0 ("y")
                      n130 = Unbundle By Name(w1114) -> ("Phasor C"=w1127:dbl, "Phasor C"=w1121:dbl, "Phasor C"=w1119:dbl)
                      n131 = Absolute Value(x=w1127) -> (abs(x)=w1128:dbl)
                      n132 = Absolute Value(x=w1121) -> (abs(x)=w1120:dbl)
                      n133 = Absolute Value(x=w1119) -> (abs(x)=w1118:dbl)
                      n134 = Multiply(x=w1128, y=w1115) -> (x*y=w1129:dbl)
                      n135 = Multiply(x=w1120, y=w1115) -> (x*y=w1124:dbl)
                      n136 = Multiply(x=w1118, y=w1115) -> (x*y=w1122:dbl)
                      n137 = Round To Nearest(number=w1129) -> (nearest integer value=w1130:dbl)
                      n138 = Round To Nearest(number=w1124) -> (nearest integer value=w1125:dbl)
                      n139 = Round To Nearest(number=w1122) -> (nearest integer value=w1123:dbl)
                      n140 = Divide(x=w1130, y=w1115) -> (x/y=w1126:dbl)
                      n141 = Divide(x=w1125, y=w1115) -> (x/y=w1117:dbl)
                      n142 = Divide(x=w1123, y=w1115) -> (x/y=w1116:dbl)
                      n143 = Bundle(w1126, w1117, w1116) -> (→"I slider 1":cluster{dbl, dbl, dbl})  [unwired: 1 in]
                    }
                    frame 2 {
                      w1131 = 1000.0 ("y")
                      n144 = Unbundle By Name(w1148) -> ("Phasor C"=w1143:dbl, "Phasor C"=w1137:dbl, "Phasor C"=w1135:dbl)
                      n145 = Absolute Value(x=w1143) -> (abs(x)=w1144:dbl)
                      n146 = Absolute Value(x=w1137) -> (abs(x)=w1136:dbl)
                      n147 = Absolute Value(x=w1135) -> (abs(x)=w1134:dbl)
                      n148 = Multiply(x=w1144, y=w1131) -> (x*y=w1145:dbl)
                      n149 = Multiply(x=w1136, y=w1131) -> (x*y=w1140:dbl)
                      n150 = Multiply(x=w1134, y=w1131) -> (x*y=w1138:dbl)
                      n151 = Round To Nearest(number=w1145) -> (nearest integer value=w1146:dbl)
                      n152 = Round To Nearest(number=w1140) -> (nearest integer value=w1141:dbl)
                      n153 = Round To Nearest(number=w1138) -> (nearest integer value=w1139:dbl)
                      n154 = Divide(x=w1146, y=w1131) -> (x/y=w1142:dbl)
                      n155 = Divide(x=w1141, y=w1131) -> (x/y=w1133:dbl)
                      n156 = Divide(x=w1139, y=w1131) -> (x/y=w1132:dbl)
                      n157 = Bundle(w1142, w1133, w1132) -> (→"I slider 2":cluster{dbl, dbl, dbl})  [unwired: 1 in]
                    }
                    frame 3 {
                      w1151 = 1000.0 ("y")
                      n158 = Unbundle By Name(w1150) -> ("Phasor C"=w1163:dbl, "Phasor C"=w1157:dbl, "Phasor C"=w1155:dbl)
                      n159 = Absolute Value(x=w1163) -> (abs(x)=w1164:dbl)
                      n160 = Absolute Value(x=w1157) -> (abs(x)=w1156:dbl)
                      n161 = Absolute Value(x=w1155) -> (abs(x)=w1154:dbl)
                      n162 = Multiply(x=w1164, y=w1151) -> (x*y=w1165:dbl)
                      n163 = Multiply(x=w1156, y=w1151) -> (x*y=w1160:dbl)
                      n164 = Multiply(x=w1154, y=w1151) -> (x*y=w1158:dbl)
                      n165 = Round To Nearest(number=w1165) -> (nearest integer value=w1166:dbl)
                      n166 = Round To Nearest(number=w1160) -> (nearest integer value=w1161:dbl)
                      n167 = Round To Nearest(number=w1158) -> (nearest integer value=w1159:dbl)
                      n168 = Divide(x=w1166, y=w1151) -> (x/y=w1162:dbl)
                      n169 = Divide(x=w1161, y=w1151) -> (x/y=w1153:dbl)
                      n170 = Divide(x=w1159, y=w1151) -> (x/y=w1152:dbl)
                      n171 = Bundle(w1162, w1153, w1152) -> (→"I slider 3":cluster{dbl, dbl, dbl})  [unwired: 1 in]
                    }
                    frame 4 {
                      w1169 = 1000.0 ("y")
                      n172 = Unbundle By Name(w1168) -> ("Phasor C"=w1181:dbl, "Phasor C"=w1175:dbl, "Phasor C"=w1173:dbl)
                      n173 = Absolute Value(x=w1181) -> (abs(x)=w1182:dbl)
                      n174 = Absolute Value(x=w1175) -> (abs(x)=w1174:dbl)
                      n175 = Absolute Value(x=w1173) -> (abs(x)=w1172:dbl)
                      n176 = Multiply(x=w1182, y=w1169) -> (x*y=w1183:dbl)
                      n177 = Multiply(x=w1174, y=w1169) -> (x*y=w1178:dbl)
                      n178 = Multiply(x=w1172, y=w1169) -> (x*y=w1176:dbl)
                      n179 = Round To Nearest(number=w1183) -> (nearest integer value=w1184:dbl)
                      n180 = Round To Nearest(number=w1178) -> (nearest integer value=w1179:dbl)
                      n181 = Round To Nearest(number=w1176) -> (nearest integer value=w1177:dbl)
                      n182 = Divide(x=w1184, y=w1169) -> (x/y=w1180:dbl)
                      n183 = Divide(x=w1179, y=w1169) -> (x/y=w1171:dbl)
                      n184 = Divide(x=w1177, y=w1169) -> (x/y=w1170:dbl)
                      n185 = Bundle(w1180, w1171, w1170) -> (→"I slider 4":cluster{dbl, dbl, dbl})  [unwired: 1 in]
                    }
                    frame 5 {
                      w1187 = 1000.0 ("y")
                      n186 = Unbundle By Name(w1186) -> ("Phasor C"=w1199:dbl, "Phasor C"=w1193:dbl, "Phasor C"=w1191:dbl)
                      n187 = Absolute Value(x=w1199) -> (abs(x)=w1200:dbl)
                      n188 = Absolute Value(x=w1193) -> (abs(x)=w1192:dbl)
                      n189 = Absolute Value(x=w1191) -> (abs(x)=w1190:dbl)
                      n190 = Multiply(x=w1200, y=w1187) -> (x*y=w1201:dbl)
                      n191 = Multiply(x=w1192, y=w1187) -> (x*y=w1196:dbl)
                      n192 = Multiply(x=w1190, y=w1187) -> (x*y=w1194:dbl)
                      n193 = Round To Nearest(number=w1201) -> (nearest integer value=w1202:dbl)
                      n194 = Round To Nearest(number=w1196) -> (nearest integer value=w1197:dbl)
                      n195 = Round To Nearest(number=w1194) -> (nearest integer value=w1195:dbl)
                      n196 = Divide(x=w1202, y=w1187) -> (x/y=w1198:dbl)
                      n197 = Divide(x=w1197, y=w1187) -> (x/y=w1189:dbl)
                      n198 = Divide(x=w1195, y=w1187) -> (x/y=w1188:dbl)
                      n199 = Bundle(w1198, w1189, w1188) -> (→"I slider 5":cluster{dbl, dbl, dbl})  [unwired: 1 in]
                    }
                    frame 6 {
                      w1203 = 1000.0 ("y")
                      n200 = Unbundle By Name(w1220) -> ("Phasor C"=w1215:dbl, "Phasor C"=w1209:dbl, "Phasor C"=w1207:dbl)
                      n201 = Absolute Value(x=w1215) -> (abs(x)=w1216:dbl)
                      n202 = Absolute Value(x=w1209) -> (abs(x)=w1208:dbl)
                      n203 = Absolute Value(x=w1207) -> (abs(x)=w1206:dbl)
                      n204 = Multiply(x=w1216, y=w1203) -> (x*y=w1217:dbl)
                      n205 = Multiply(x=w1208, y=w1203) -> (x*y=w1212:dbl)
                      n206 = Multiply(x=w1206, y=w1203) -> (x*y=w1210:dbl)
                      n207 = Round To Nearest(number=w1217) -> (nearest integer value=w1218:dbl)
                      n208 = Round To Nearest(number=w1212) -> (nearest integer value=w1213:dbl)
                      n209 = Round To Nearest(number=w1210) -> (nearest integer value=w1211:dbl)
                      n210 = Divide(x=w1218, y=w1203) -> (x/y=w1214:dbl)
                      n211 = Divide(x=w1213, y=w1203) -> (x/y=w1205:dbl)
                      n212 = Divide(x=w1211, y=w1203) -> (x/y=w1204:dbl)
                      n213 = Bundle(w1214, w1205, w1204) -> (→"I slider 6":cluster{dbl, dbl, dbl})  [unwired: 1 in]
                    }
                    frame 7 {
                      w1223 = 1000.0 ("y")
                      n214 = Unbundle By Name(w1222) -> ("Phasor C"=w1235:dbl, "Phasor C"=w1229:dbl, "Phasor C"=w1227:dbl)
                      n215 = Absolute Value(x=w1235) -> (abs(x)=w1236:dbl)
                      n216 = Absolute Value(x=w1229) -> (abs(x)=w1228:dbl)
                      n217 = Absolute Value(x=w1227) -> (abs(x)=w1226:dbl)
                      n218 = Multiply(x=w1236, y=w1223) -> (x*y=w1237:dbl)
                      n219 = Multiply(x=w1228, y=w1223) -> (x*y=w1232:dbl)
                      n220 = Multiply(x=w1226, y=w1223) -> (x*y=w1230:dbl)
                      n221 = Round To Nearest(number=w1237) -> (nearest integer value=w1238:dbl)
                      n222 = Round To Nearest(number=w1232) -> (nearest integer value=w1233:dbl)
                      n223 = Round To Nearest(number=w1230) -> (nearest integer value=w1231:dbl)
                      n224 = Divide(x=w1238, y=w1223) -> (x/y=w1234:dbl)
                      n225 = Divide(x=w1233, y=w1223) -> (x/y=w1225:dbl)
                      n226 = Divide(x=w1231, y=w1223) -> (x/y=w1224:dbl)
                      n227 = Bundle(w1234, w1225, w1224) -> (→"I slider 7":cluster{dbl, dbl, dbl})  [unwired: 1 in]
                    }
                    frame 8 {
                      w1239 = 1000.0 ("y")
                      n228 = Unbundle By Name(w1256) -> ("Phasor C"=w1251:dbl, "Phasor C"=w1245:dbl, "Phasor C"=w1243:dbl)
                      n229 = Absolute Value(x=w1251) -> (abs(x)=w1252:dbl)
                      n230 = Absolute Value(x=w1245) -> (abs(x)=w1244:dbl)
                      n231 = Absolute Value(x=w1243) -> (abs(x)=w1242:dbl)
                      n232 = Multiply(x=w1252, y=w1239) -> (x*y=w1253:dbl)
                      n233 = Multiply(x=w1244, y=w1239) -> (x*y=w1248:dbl)
                      n234 = Multiply(x=w1242, y=w1239) -> (x*y=w1246:dbl)
                      n235 = Round To Nearest(number=w1253) -> (nearest integer value=w1254:dbl)
                      n236 = Round To Nearest(number=w1248) -> (nearest integer value=w1249:dbl)
                      n237 = Round To Nearest(number=w1246) -> (nearest integer value=w1247:dbl)
                      n238 = Divide(x=w1254, y=w1239) -> (x/y=w1250:dbl)
                      n239 = Divide(x=w1249, y=w1239) -> (x/y=w1241:dbl)
                      n240 = Divide(x=w1247, y=w1239) -> (x/y=w1240:dbl)
                      n241 = Bundle(w1250, w1241, w1240) -> (→"I slider 8":cluster{dbl, dbl, dbl})  [unwired: 1 in]
                    }
                    frame 9 {
                      w1259 = 1000.0 ("y")
                      n242 = Unbundle By Name(w1258) -> ("Phasor C"=w1271:dbl, "Phasor C"=w1265:dbl, "Phasor C"=w1263:dbl)
                      n243 = Absolute Value(x=w1271) -> (abs(x)=w1272:dbl)
                      n244 = Absolute Value(x=w1265) -> (abs(x)=w1264:dbl)
                      n245 = Absolute Value(x=w1263) -> (abs(x)=w1262:dbl)
                      n246 = Multiply(x=w1272, y=w1259) -> (x*y=w1273:dbl)
                      n247 = Multiply(x=w1264, y=w1259) -> (x*y=w1268:dbl)
                      n248 = Multiply(x=w1262, y=w1259) -> (x*y=w1266:dbl)
                      n249 = Round To Nearest(number=w1273) -> (nearest integer value=w1274:dbl)
                      n250 = Round To Nearest(number=w1268) -> (nearest integer value=w1269:dbl)
                      n251 = Round To Nearest(number=w1266) -> (nearest integer value=w1267:dbl)
                      n252 = Divide(x=w1274, y=w1259) -> (x/y=w1270:dbl)
                      n253 = Divide(x=w1269, y=w1259) -> (x/y=w1261:dbl)
                      n254 = Divide(x=w1267, y=w1259) -> (x/y=w1260:dbl)
                      n255 = Bundle(w1270, w1261, w1260) -> (→"I slider 9":cluster{dbl, dbl, dbl})  [unwired: 1 in]
                    }
                    frame 10 {
                      w1275 = 1000.0 ("y")
                      n256 = Unbundle By Name(w1292) -> ("Phasor C"=w1287:dbl, "Phasor C"=w1281:dbl, "Phasor C"=w1279:dbl)
                      n257 = Absolute Value(x=w1287) -> (abs(x)=w1288:dbl)
                      n258 = Absolute Value(x=w1281) -> (abs(x)=w1280:dbl)
                      n259 = Absolute Value(x=w1279) -> (abs(x)=w1278:dbl)
                      n260 = Multiply(x=w1288, y=w1275) -> (x*y=w1289:dbl)
                      n261 = Multiply(x=w1280, y=w1275) -> (x*y=w1284:dbl)
                      n262 = Multiply(x=w1278, y=w1275) -> (x*y=w1282:dbl)
                      n263 = Round To Nearest(number=w1289) -> (nearest integer value=w1290:dbl)
                      n264 = Round To Nearest(number=w1284) -> (nearest integer value=w1285:dbl)
                      n265 = Round To Nearest(number=w1282) -> (nearest integer value=w1283:dbl)
                      n266 = Divide(x=w1290, y=w1275) -> (x/y=w1286:dbl)
                      n267 = Divide(x=w1285, y=w1275) -> (x/y=w1277:dbl)
                      n268 = Divide(x=w1283, y=w1275) -> (x/y=w1276:dbl)
                      n269 = Bundle(w1286, w1277, w1276) -> (→"I slider 10":cluster{dbl, dbl, dbl})  [unwired: 1 in]
                    }
                    frame 11 {
                      w1295 = 1000.0 ("y")
                      n270 = Unbundle By Name(w1294) -> ("Phasor C"=w1307:dbl, "Phasor C"=w1301:dbl, "Phasor C"=w1299:dbl)
                      n271 = Absolute Value(x=w1307) -> (abs(x)=w1308:dbl)
                      n272 = Absolute Value(x=w1301) -> (abs(x)=w1300:dbl)
                      n273 = Absolute Value(x=w1299) -> (abs(x)=w1298:dbl)
                      n274 = Multiply(x=w1308, y=w1295) -> (x*y=w1309:dbl)
                      n275 = Multiply(x=w1300, y=w1295) -> (x*y=w1304:dbl)
                      n276 = Multiply(x=w1298, y=w1295) -> (x*y=w1302:dbl)
                      n277 = Round To Nearest(number=w1309) -> (nearest integer value=w1310:dbl)
                      n278 = Round To Nearest(number=w1304) -> (nearest integer value=w1305:dbl)
                      n279 = Round To Nearest(number=w1302) -> (nearest integer value=w1303:dbl)
                      n280 = Divide(x=w1310, y=w1295) -> (x/y=w1306:dbl)
                      n281 = Divide(x=w1305, y=w1295) -> (x/y=w1297:dbl)
                      n282 = Divide(x=w1303, y=w1295) -> (x/y=w1296:dbl)
                      n283 = Bundle(w1306, w1297, w1296) -> (→"I slider 11":cluster{dbl, dbl, dbl})  [unwired: 1 in]
                    }
                    frame 12 {
                      w1313 = 1000.0 ("y")
                      n284 = Unbundle By Name(w1312) -> ("Phasor C"=w1325:dbl, "Phasor C"=w1319:dbl, "Phasor C"=w1317:dbl)
                      n285 = Absolute Value(x=w1325) -> (abs(x)=w1326:dbl)
                      n286 = Absolute Value(x=w1319) -> (abs(x)=w1318:dbl)
                      n287 = Absolute Value(x=w1317) -> (abs(x)=w1316:dbl)
                      n288 = Multiply(x=w1326, y=w1313) -> (x*y=w1327:dbl)
                      n289 = Multiply(x=w1318, y=w1313) -> (x*y=w1322:dbl)
                      n290 = Multiply(x=w1316, y=w1313) -> (x*y=w1320:dbl)
                      n291 = Round To Nearest(number=w1327) -> (nearest integer value=w1328:dbl)
                      n292 = Round To Nearest(number=w1322) -> (nearest integer value=w1323:dbl)
                      n293 = Round To Nearest(number=w1320) -> (nearest integer value=w1321:dbl)
                      n294 = Divide(x=w1328, y=w1313) -> (x/y=w1324:dbl)
                      n295 = Divide(x=w1323, y=w1313) -> (x/y=w1315:dbl)
                      n296 = Divide(x=w1321, y=w1313) -> (x/y=w1314:dbl)
                      n297 = Bundle(w1324, w1315, w1314) -> (→"I slider 12":cluster{dbl, dbl, dbl})  [unwired: 1 in]
                    }
                    frame 13 {
                      w1331 = 1000.0 ("y")
                      n298 = Unbundle By Name(w1330) -> ("Phasor C"=w1343:dbl, "Phasor C"=w1337:dbl, "Phasor C"=w1335:dbl)
                      n299 = Absolute Value(x=w1343) -> (abs(x)=w1344:dbl)
                      n300 = Absolute Value(x=w1337) -> (abs(x)=w1336:dbl)
                      n301 = Absolute Value(x=w1335) -> (abs(x)=w1334:dbl)
                      n302 = Multiply(x=w1344, y=w1331) -> (x*y=w1345:dbl)
                      n303 = Multiply(x=w1336, y=w1331) -> (x*y=w1340:dbl)
                      n304 = Multiply(x=w1334, y=w1331) -> (x*y=w1338:dbl)
                      n305 = Round To Nearest(number=w1345) -> (nearest integer value=w1346:dbl)
                      n306 = Round To Nearest(number=w1340) -> (nearest integer value=w1341:dbl)
                      n307 = Round To Nearest(number=w1338) -> (nearest integer value=w1339:dbl)
                      n308 = Divide(x=w1346, y=w1331) -> (x/y=w1342:dbl)
                      n309 = Divide(x=w1341, y=w1331) -> (x/y=w1333:dbl)
                      n310 = Divide(x=w1339, y=w1331) -> (x/y=w1332:dbl)
                      n311 = Bundle(w1342, w1333, w1332) -> (→"I slider 13":cluster{dbl, dbl, dbl})  [unwired: 1 in]
                    }
                    frame 14 {
                      w1349 = 1000.0 ("y")
                      n312 = Unbundle By Name(w1348) -> ("Phasor C"=w1361:dbl, "Phasor C"=w1355:dbl, "Phasor C"=w1353:dbl)
                      n313 = Absolute Value(x=w1361) -> (abs(x)=w1362:dbl)
                      n314 = Absolute Value(x=w1355) -> (abs(x)=w1354:dbl)
                      n315 = Absolute Value(x=w1353) -> (abs(x)=w1352:dbl)
                      n316 = Multiply(x=w1362, y=w1349) -> (x*y=w1363:dbl)
                      n317 = Multiply(x=w1354, y=w1349) -> (x*y=w1358:dbl)
                      n318 = Multiply(x=w1352, y=w1349) -> (x*y=w1356:dbl)
                      n319 = Round To Nearest(number=w1363) -> (nearest integer value=w1364:dbl)
                      n320 = Round To Nearest(number=w1358) -> (nearest integer value=w1359:dbl)
                      n321 = Round To Nearest(number=w1356) -> (nearest integer value=w1357:dbl)
                      n322 = Divide(x=w1364, y=w1349) -> (x/y=w1360:dbl)
                      n323 = Divide(x=w1359, y=w1349) -> (x/y=w1351:dbl)
                      n324 = Divide(x=w1357, y=w1349) -> (x/y=w1350:dbl)
                      n325 = Bundle(w1360, w1351, w1350) -> (→"I slider 14":cluster{dbl, dbl, dbl})  [unwired: 1 in]
                    }
                    frame 15 {
                      w1367 = 1000.0 ("y")
                      n326 = Unbundle By Name(w1366) -> ("Phasor C"=w1379:dbl, "Phasor C"=w1373:dbl, "Phasor C"=w1371:dbl)
                      n327 = Absolute Value(x=w1379) -> (abs(x)=w1380:dbl)
                      n328 = Absolute Value(x=w1373) -> (abs(x)=w1372:dbl)
                      n329 = Absolute Value(x=w1371) -> (abs(x)=w1370:dbl)
                      n330 = Multiply(x=w1380, y=w1367) -> (x*y=w1381:dbl)
                      n331 = Multiply(x=w1372, y=w1367) -> (x*y=w1376:dbl)
                      n332 = Multiply(x=w1370, y=w1367) -> (x*y=w1374:dbl)
                      n333 = Round To Nearest(number=w1381) -> (nearest integer value=w1382:dbl)
                      n334 = Round To Nearest(number=w1376) -> (nearest integer value=w1377:dbl)
                      n335 = Round To Nearest(number=w1374) -> (nearest integer value=w1375:dbl)
                      n336 = Divide(x=w1382, y=w1367) -> (x/y=w1378:dbl)
                      n337 = Divide(x=w1377, y=w1367) -> (x/y=w1369:dbl)
                      n338 = Divide(x=w1375, y=w1367) -> (x/y=w1368:dbl)
                      n339 = Bundle(w1378, w1369, w1368) -> (→"I slider 15":cluster{dbl, dbl, dbl})  [unwired: 1 in]
                    }
                    frame 16 {
                      w1385 = 1000.0 ("y")
                      n340 = Unbundle By Name(w1384) -> ("Phasor C"=w1397:dbl, "Phasor C"=w1391:dbl, "Phasor C"=w1389:dbl)
                      n341 = Absolute Value(x=w1397) -> (abs(x)=w1398:dbl)
                      n342 = Absolute Value(x=w1391) -> (abs(x)=w1390:dbl)
                      n343 = Absolute Value(x=w1389) -> (abs(x)=w1388:dbl)
                      n344 = Multiply(x=w1398, y=w1385) -> (x*y=w1399:dbl)
                      n345 = Multiply(x=w1390, y=w1385) -> (x*y=w1394:dbl)
                      n346 = Multiply(x=w1388, y=w1385) -> (x*y=w1392:dbl)
                      n347 = Round To Nearest(number=w1399) -> (nearest integer value=w1400:dbl)
                      n348 = Round To Nearest(number=w1394) -> (nearest integer value=w1395:dbl)
                      n349 = Round To Nearest(number=w1392) -> (nearest integer value=w1393:dbl)
                      n350 = Divide(x=w1400, y=w1385) -> (x/y=w1396:dbl)
                      n351 = Divide(x=w1395, y=w1385) -> (x/y=w1387:dbl)
                      n352 = Divide(x=w1393, y=w1385) -> (x/y=w1386:dbl)
                      n353 = Bundle(w1396, w1387, w1386) -> (→"I slider 16":cluster{dbl, dbl, dbl})  [unwired: 1 in]
                    }
                    frame 17 {
                      w1401 = 1000.0 ("y")
                      n354 = Unbundle By Name(w1403) -> ("Phasor C"=w1404:dbl)
                      n355 = Absolute Value(x=w1404) -> (abs(x)=w1405:dbl)
                      n356 = Multiply(x=w1405, y=w1401) -> (x*y=w1406:dbl)
                      n357 = Round To Nearest(number=w1406) -> (nearest integer value=w1407:dbl)
                      n358 = Divide(x=w1407, y=w1401) -> (x/y=→"I slider 17":dbl)
                    }
                    frame 18 {
                      w1408 = 1000.0 ("y")
                      n359 = Unbundle By Name(w1410) -> ("Phasor C"=w1411:dbl)
                      n360 = Absolute Value(x=w1411) -> (abs(x)=w1412:dbl)
                      n361 = Multiply(x=w1412, y=w1408) -> (x*y=w1413:dbl)
                      n362 = Round To Nearest(number=w1413) -> (nearest integer value=w1414:dbl)
                      n363 = Divide(x=w1414, y=w1408) -> (x/y=→"I slider 18":dbl)
                    }
                    frame 19 {
                      w1415 = 1000.0 ("y")
                      n364 = Unbundle By Name(w1417) -> ("Phasor C"=w1418:dbl)
                      n365 = Absolute Value(x=w1418) -> (abs(x)=w1419:dbl)
                      n366 = Multiply(x=w1419, y=w1415) -> (x*y=w1420:dbl)
                      n367 = Round To Nearest(number=w1420) -> (nearest integer value=w1421:dbl)
                      n368 = Divide(x=w1421, y=w1415) -> (x/y=→"I slider 19":dbl)
                    }
                    frame 20 {
                      w1422 = 1000.0 ("y")
                      n369 = Unbundle By Name(w1424) -> ("Phasor C"=w1425:dbl)
                      n370 = Absolute Value(x=w1425) -> (abs(x)=w1426:dbl)
                      n371 = Multiply(x=w1426, y=w1422) -> (x*y=w1427:dbl)
                      n372 = Round To Nearest(number=w1427) -> (nearest integer value=w1428:dbl)
                      n373 = Divide(x=w1428, y=w1422) -> (x/y=→"I slider 20":dbl)
                    }
                    frame 21, Default {
                    }
                  }
                }
              }
            }
            n374 = for {
              tunnel: w454 -> [w673] mode=indexing
              i -> [w672]
              n375 = Unbundle By Name(w673) -> ("Iinjected"=w671:cdb[], "Sinjected"=w670:cdb[])
              n376 = case shown="True" TRUE {
                tunnel: w672 -> [_ w676]
                tunnel: w670 -> [_ w675]
                tunnel: w671 -> [_ w674]
                frame False {
                }
                frame True {
                  n377 = case shown="2" w676 {
                    tunnel: w674 -> [_ w695 w710 w729 w744 w763 w778 w793 w808 w827 w842 w861 w876 w895 w914 w933 w952 w971 w990 w993 w1005 w1017 w1029 w1041 w1053 w1065 w1077]
                    tunnel: w675 -> [_ w694 w709 w728 w743 w762 w777 w792 w807 w826 w841 w860 w875 w894 w913 w932 w951 w970 w989 w995 w1007 w1019 w1031 w1043 w1055 w1067 w1079]
                    frame 100, Default {
                    }
                    frame 0 {
                      w677 = 1000.0 ("y")
                      n378 = Complex To Re/Im(x + iy=w694) -> (x=w693:dbl[], y=w692:dbl[])
                      n379 = Absolute Value(x=w695) -> (abs(x)=w691:dbl[])
                      n380 = Add Array Elements(numeric array=w691) -> (sum=w690:dbl)
                      n381 = Add Array Elements(numeric array=w693) -> (sum=w684:dbl)
                      n382 = Add Array Elements(numeric array=w692) -> (sum=w686:dbl)
                      n383 = Divide(x=w690, y=3.0) -> (x/y=w678:dbl)
                      n384 = Round To Nearest(number=w684) -> (nearest integer value=w683:dbl)
                      n385 = Round To Nearest(number=w686) -> (nearest integer value=w685:dbl)
                      n386 = Multiply(x=w678, y=w677) -> (x*y=w679:dbl)
                      n387 = Round To Nearest(number=w679) -> (nearest integer value=w680:dbl)
                      n388 = Divide(x=w683, y=w677) -> (x/y=→"kW":dbl)
                      n389 = Divide(x=w685, y=w677) -> (x/y=→"?VkVAr":dbl)
                      n390 = Divide(x=w680, y=w677) -> (x/y=w681:dbl)
                      n391 = node(w681) -> (→"A":dbl[unit])
                    }
                    frame 1 {
                      w696 = 1000.0 ("y")
                      n392 = Complex To Re/Im(x + iy=w709) -> (x=w708:dbl[], y=w707:dbl[])
                      n393 = Absolute Value(x=w710) -> (abs(x)=w706:dbl[])
                      n394 = Add Array Elements(numeric array=w706) -> (sum=w705:dbl)
                      n395 = Add Array Elements(numeric array=w708) -> (sum=w701:dbl)
                      n396 = Add Array Elements(numeric array=w707) -> (sum=w703:dbl)
                      n397 = Divide(x=w705, y=3.0) -> (x/y=w697:dbl)
                      n398 = Round To Nearest(number=w701) -> (nearest integer value=w700:dbl)
                      n399 = Round To Nearest(number=w703) -> (nearest integer value=w702:dbl)
                      n400 = Multiply(x=w697, y=w696) -> (x*y=w698:dbl)
                      n401 = Round To Nearest(number=w698) -> (nearest integer value=w699:dbl)
                      n402 = Divide(x=w700, y=w696) -> ()  [unwired: 1 out]
                      n403 = Divide(x=w702, y=w696) -> ()  [unwired: 1 out]
                      n404 = Divide(x=w699, y=w696) -> ()  [unwired: 1 out]
                    }
                    frame 2 {
                      w711 = 1000.0 ("y")
                      n405 = Complex To Re/Im(x + iy=w728) -> (x=w727:dbl[], y=w726:dbl[])
                      n406 = Absolute Value(x=w729) -> (abs(x)=w725:dbl[])
                      n407 = Add Array Elements(numeric array=w725) -> (sum=w724:dbl)
                      n408 = Add Array Elements(numeric array=w727) -> (sum=w718:dbl)
                      n409 = Add Array Elements(numeric array=w726) -> (sum=w720:dbl)
                      n410 = Divide(x=w724, y=3.0) -> (x/y=w712:dbl)
                      n411 = Round To Nearest(number=w718) -> (nearest integer value=w717:dbl)
                      n412 = Round To Nearest(number=w720) -> (nearest integer value=w719:dbl)
                      n413 = Multiply(x=w712, y=w711) -> (x*y=w713:dbl)
                      n414 = Round To Nearest(number=w713) -> (nearest integer value=w714:dbl)
                      n415 = Divide(x=w717, y=w711) -> (x/y=→"kW":dbl)
                      n416 = Divide(x=w719, y=w711) -> (x/y=→"?VkVAr":dbl)
                      n417 = Divide(x=w714, y=w711) -> (x/y=w715:dbl)
                      n418 = node(w715) -> (→"A2":dbl[unit])
                    }
                    frame 3 {
                      w730 = 1000.0 ("y")
                      n419 = Complex To Re/Im(x + iy=w743) -> (x=w742:dbl[], y=w741:dbl[])
                      n420 = Absolute Value(x=w744) -> (abs(x)=w740:dbl[])
                      n421 = Add Array Elements(numeric array=w740) -> (sum=w739:dbl)
                      n422 = Add Array Elements(numeric array=w742) -> (sum=w735:dbl)
                      n423 = Add Array Elements(numeric array=w741) -> (sum=w737:dbl)
                      n424 = Divide(x=w739, y=3.0) -> (x/y=w731:dbl)
                      n425 = Round To Nearest(number=w735) -> (nearest integer value=w734:dbl)
                      n426 = Round To Nearest(number=w737) -> (nearest integer value=w736:dbl)
                      n427 = Multiply(x=w731, y=w730) -> (x*y=w732:dbl)
                      n428 = Round To Nearest(number=w732) -> (nearest integer value=w733:dbl)
                      n429 = Divide(x=w734, y=w730) -> ()  [unwired: 1 out]
                      n430 = Divide(x=w736, y=w730) -> ()  [unwired: 1 out]
                      n431 = Divide(x=w733, y=w730) -> ()  [unwired: 1 out]
                    }
                    frame 4 {
                      w745 = 1000.0 ("y")
                      n432 = Complex To Re/Im(x + iy=w762) -> (x=w761:dbl[], y=w760:dbl[])
                      n433 = Absolute Value(x=w763) -> (abs(x)=w759:dbl[])
                      n434 = Add Array Elements(numeric array=w759) -> (sum=w758:dbl)
                      n435 = Add Array Elements(numeric array=w761) -> (sum=w752:dbl)
                      n436 = Add Array Elements(numeric array=w760) -> (sum=w754:dbl)
                      n437 = Divide(x=w758, y=3.0) -> (x/y=w746:dbl)
                      n438 = Round To Nearest(number=w752) -> (nearest integer value=w751:dbl)
                      n439 = Round To Nearest(number=w754) -> (nearest integer value=w753:dbl)
                      n440 = Multiply(x=w746, y=w745) -> (x*y=w747:dbl)
                      n441 = Round To Nearest(number=w747) -> (nearest integer value=w748:dbl)
                      n442 = Divide(x=w751, y=w745) -> (x/y=→"kW":dbl)
                      n443 = Divide(x=w753, y=w745) -> (x/y=→"?VkVAr":dbl)
                      n444 = Divide(x=w748, y=w745) -> (x/y=w749:dbl)
                      n445 = node(w749) -> (→"A":dbl[unit])
                    }
                    frame 5 {
                      w764 = 1000.0 ("y")
                      n446 = Complex To Re/Im(x + iy=w777) -> (x=w776:dbl[], y=w775:dbl[])
                      n447 = Absolute Value(x=w778) -> (abs(x)=w774:dbl[])
                      n448 = Add Array Elements(numeric array=w774) -> (sum=w773:dbl)
                      n449 = Add Array Elements(numeric array=w776) -> (sum=w769:dbl)
                      n450 = Add Array Elements(numeric array=w775) -> (sum=w771:dbl)
                      n451 = Divide(x=w773, y=3.0) -> (x/y=w765:dbl)
                      n452 = Round To Nearest(number=w769) -> (nearest integer value=w768:dbl)
                      n453 = Round To Nearest(number=w771) -> (nearest integer value=w770:dbl)
                      n454 = Multiply(x=w765, y=w764) -> (x*y=w766:dbl)
                      n455 = Round To Nearest(number=w766) -> (nearest integer value=w767:dbl)
                      n456 = Divide(x=w768, y=w764) -> ()  [unwired: 1 out]
                      n457 = Divide(x=w770, y=w764) -> ()  [unwired: 1 out]
                      n458 = Divide(x=w767, y=w764) -> ()  [unwired: 1 out]
                    }
                    frame 6 {
                      w779 = 1000.0 ("y")
                      n459 = Complex To Re/Im(x + iy=w792) -> (x=w791:dbl[], y=w790:dbl[])
                      n460 = Absolute Value(x=w793) -> (abs(x)=w789:dbl[])
                      n461 = Add Array Elements(numeric array=w789) -> (sum=w788:dbl)
                      n462 = Add Array Elements(numeric array=w791) -> (sum=w784:dbl)
                      n463 = Add Array Elements(numeric array=w790) -> (sum=w786:dbl)
                      n464 = Divide(x=w788, y=3.0) -> (x/y=w780:dbl)
                      n465 = Round To Nearest(number=w784) -> (nearest integer value=w783:dbl)
                      n466 = Round To Nearest(number=w786) -> (nearest integer value=w785:dbl)
                      n467 = Multiply(x=w780, y=w779) -> (x*y=w781:dbl)
                      n468 = Round To Nearest(number=w781) -> (nearest integer value=w782:dbl)
                      n469 = Divide(x=w783, y=w779) -> ()  [unwired: 1 out]
                      n470 = Divide(x=w785, y=w779) -> ()  [unwired: 1 out]
                      n471 = Divide(x=w782, y=w779) -> ()  [unwired: 1 out]
                    }
                    frame 7 {
                      w794 = 1000.0 ("y")
                      n472 = Complex To Re/Im(x + iy=w807) -> (x=w806:dbl[], y=w805:dbl[])
                      n473 = Absolute Value(x=w808) -> (abs(x)=w804:dbl[])
                      n474 = Add Array Elements(numeric array=w804) -> (sum=w803:dbl)
                      n475 = Add Array Elements(numeric array=w806) -> (sum=w799:dbl)
                      n476 = Add Array Elements(numeric array=w805) -> (sum=w801:dbl)
                      n477 = Divide(x=w803, y=3.0) -> (x/y=w795:dbl)
                      n478 = Round To Nearest(number=w799) -> (nearest integer value=w798:dbl)
                      n479 = Round To Nearest(number=w801) -> (nearest integer value=w800:dbl)
                      n480 = Multiply(x=w795, y=w794) -> (x*y=w796:dbl)
                      n481 = Round To Nearest(number=w796) -> (nearest integer value=w797:dbl)
                      n482 = Divide(x=w798, y=w794) -> ()  [unwired: 1 out]
                      n483 = Divide(x=w800, y=w794) -> ()  [unwired: 1 out]
                      n484 = Divide(x=w797, y=w794) -> ()  [unwired: 1 out]
                    }
                    frame 8 {
                      w809 = 1000.0 ("y")
                      n485 = Complex To Re/Im(x + iy=w826) -> (x=w825:dbl[], y=w824:dbl[])
                      n486 = Absolute Value(x=w827) -> (abs(x)=w823:dbl[])
                      n487 = Add Array Elements(numeric array=w823) -> (sum=w822:dbl)
                      n488 = Add Array Elements(numeric array=w825) -> (sum=w816:dbl)
                      n489 = Add Array Elements(numeric array=w824) -> (sum=w818:dbl)
                      n490 = Divide(x=w822, y=3.0) -> (x/y=w810:dbl)
                      n491 = Round To Nearest(number=w816) -> (nearest integer value=w815:dbl)
                      n492 = Round To Nearest(number=w818) -> (nearest integer value=w817:dbl)
                      n493 = Multiply(x=w810, y=w809) -> (x*y=w811:dbl)
                      n494 = Round To Nearest(number=w811) -> (nearest integer value=w812:dbl)
                      n495 = Divide(x=w815, y=w809) -> (x/y=→"kW":dbl)
                      n496 = Divide(x=w817, y=w809) -> (x/y=→"?VkVAr":dbl)
                      n497 = Divide(x=w812, y=w809) -> (x/y=w813:dbl)
                      n498 = node(w813) -> (→"A":dbl[unit])
                    }
                    frame 9 {
                      w828 = 1000.0 ("y")
                      n499 = Complex To Re/Im(x + iy=w841) -> (x=w840:dbl[], y=w839:dbl[])
                      n500 = Absolute Value(x=w842) -> (abs(x)=w838:dbl[])
                      n501 = Add Array Elements(numeric array=w838) -> (sum=w837:dbl)
                      n502 = Add Array Elements(numeric array=w840) -> (sum=w833:dbl)
                      n503 = Add Array Elements(numeric array=w839) -> (sum=w835:dbl)
                      n504 = Divide(x=w837, y=3.0) -> (x/y=w829:dbl)
                      n505 = Round To Nearest(number=w833) -> (nearest integer value=w832:dbl)
                      n506 = Round To Nearest(number=w835) -> (nearest integer value=w834:dbl)
                      n507 = Multiply(x=w829, y=w828) -> (x*y=w830:dbl)
                      n508 = Round To Nearest(number=w830) -> (nearest integer value=w831:dbl)
                      n509 = Divide(x=w832, y=w828) -> ()  [unwired: 1 out]
                      n510 = Divide(x=w834, y=w828) -> ()  [unwired: 1 out]
                      n511 = Divide(x=w831, y=w828) -> ()  [unwired: 1 out]
                    }
                    frame 10 {
                      w843 = 1000.0 ("y")
                      n512 = Complex To Re/Im(x + iy=w860) -> (x=w859:dbl[], y=w858:dbl[])
                      n513 = Absolute Value(x=w861) -> (abs(x)=w857:dbl[])
                      n514 = Add Array Elements(numeric array=w857) -> (sum=w856:dbl)
                      n515 = Add Array Elements(numeric array=w859) -> (sum=w850:dbl)
                      n516 = Add Array Elements(numeric array=w858) -> (sum=w852:dbl)
                      n517 = Divide(x=w856, y=3.0) -> (x/y=w844:dbl)
                      n518 = Round To Nearest(number=w850) -> (nearest integer value=w849:dbl)
                      n519 = Round To Nearest(number=w852) -> (nearest integer value=w851:dbl)
                      n520 = Multiply(x=w844, y=w843) -> (x*y=w845:dbl)
                      n521 = Round To Nearest(number=w845) -> (nearest integer value=w846:dbl)
                      n522 = Divide(x=w849, y=w843) -> (x/y=→"kW":dbl)
                      n523 = Divide(x=w851, y=w843) -> (x/y=→"?VkVAr":dbl)
                      n524 = Divide(x=w846, y=w843) -> (x/y=w847:dbl)
                      n525 = node(w847) -> (→"A":dbl[unit])
                    }
                    frame 11 {
                      w862 = 1000.0 ("y")
                      n526 = Complex To Re/Im(x + iy=w875) -> (x=w874:dbl[], y=w873:dbl[])
                      n527 = Absolute Value(x=w876) -> (abs(x)=w872:dbl[])
                      n528 = Add Array Elements(numeric array=w872) -> (sum=w871:dbl)
                      n529 = Add Array Elements(numeric array=w874) -> (sum=w867:dbl)
                      n530 = Add Array Elements(numeric array=w873) -> (sum=w869:dbl)
                      n531 = Divide(x=w871, y=3.0) -> (x/y=w863:dbl)
                      n532 = Round To Nearest(number=w867) -> (nearest integer value=w866:dbl)
                      n533 = Round To Nearest(number=w869) -> (nearest integer value=w868:dbl)
                      n534 = Multiply(x=w863, y=w862) -> (x*y=w864:dbl)
                      n535 = Round To Nearest(number=w864) -> (nearest integer value=w865:dbl)
                      n536 = Divide(x=w866, y=w862) -> ()  [unwired: 1 out]
                      n537 = Divide(x=w868, y=w862) -> ()  [unwired: 1 out]
                      n538 = Divide(x=w865, y=w862) -> ()  [unwired: 1 out]
                    }
                    frame 12 {
                      w877 = 1000.0 ("y")
                      n539 = Complex To Re/Im(x + iy=w894) -> (x=w893:dbl[], y=w892:dbl[])
                      n540 = Absolute Value(x=w895) -> (abs(x)=w891:dbl[])
                      n541 = Add Array Elements(numeric array=w891) -> (sum=w890:dbl)
                      n542 = Add Array Elements(numeric array=w893) -> (sum=w884:dbl)
                      n543 = Add Array Elements(numeric array=w892) -> (sum=w886:dbl)
                      n544 = Divide(x=w890, y=3.0) -> (x/y=w878:dbl)
                      n545 = Round To Nearest(number=w884) -> (nearest integer value=w883:dbl)
                      n546 = Round To Nearest(number=w886) -> (nearest integer value=w885:dbl)
                      n547 = Multiply(x=w878, y=w877) -> (x*y=w879:dbl)
                      n548 = Round To Nearest(number=w879) -> (nearest integer value=w880:dbl)
                      n549 = Divide(x=w883, y=w877) -> (x/y=→"kW":dbl)
                      n550 = Divide(x=w885, y=w877) -> (x/y=→"?VkVAr":dbl)
                      n551 = Divide(x=w880, y=w877) -> (x/y=w881:dbl)
                      n552 = node(w881) -> (→"A":dbl[unit])
                    }
                    frame 13 {
                      w896 = 1000.0 ("y")
                      n553 = Complex To Re/Im(x + iy=w913) -> (x=w912:dbl[], y=w911:dbl[])
                      n554 = Absolute Value(x=w914) -> (abs(x)=w910:dbl[])
                      n555 = Add Array Elements(numeric array=w910) -> (sum=w909:dbl)
                      n556 = Add Array Elements(numeric array=w912) -> (sum=w903:dbl)
                      n557 = Add Array Elements(numeric array=w911) -> (sum=w905:dbl)
                      n558 = Divide(x=w909, y=3.0) -> (x/y=w897:dbl)
                      n559 = Round To Nearest(number=w903) -> (nearest integer value=w902:dbl)
                      n560 = Round To Nearest(number=w905) -> (nearest integer value=w904:dbl)
                      n561 = Multiply(x=w897, y=w896) -> (x*y=w898:dbl)
                      n562 = Round To Nearest(number=w898) -> (nearest integer value=w899:dbl)
                      n563 = Divide(x=w902, y=w896) -> (x/y=→"kW":dbl)
                      n564 = Divide(x=w904, y=w896) -> (x/y=→"?VkVAr":dbl)
                      n565 = Divide(x=w899, y=w896) -> (x/y=w900:dbl)
                      n566 = node(w900) -> (→"A":dbl[unit])
                    }
                    frame 14 {
                      w915 = 1000.0 ("y")
                      n567 = Complex To Re/Im(x + iy=w932) -> (x=w931:dbl[], y=w930:dbl[])
                      n568 = Absolute Value(x=w933) -> (abs(x)=w929:dbl[])
                      n569 = Add Array Elements(numeric array=w929) -> (sum=w928:dbl)
                      n570 = Add Array Elements(numeric array=w931) -> (sum=w922:dbl)
                      n571 = Add Array Elements(numeric array=w930) -> (sum=w924:dbl)
                      n572 = Divide(x=w928, y=3.0) -> (x/y=w916:dbl)
                      n573 = Round To Nearest(number=w922) -> (nearest integer value=w921:dbl)
                      n574 = Round To Nearest(number=w924) -> (nearest integer value=w923:dbl)
                      n575 = Multiply(x=w916, y=w915) -> (x*y=w917:dbl)
                      n576 = Round To Nearest(number=w917) -> (nearest integer value=w918:dbl)
                      n577 = Divide(x=w921, y=w915) -> (x/y=→"kW":dbl)
                      n578 = Divide(x=w923, y=w915) -> (x/y=→"?VkVAr":dbl)
                      n579 = Divide(x=w918, y=w915) -> (x/y=w919:dbl)
                      n580 = node(w919) -> (→"A":dbl[unit])
                    }
                    frame 15 {
                      w934 = 1000.0 ("y")
                      n581 = Complex To Re/Im(x + iy=w951) -> (x=w950:dbl[], y=w949:dbl[])
                      n582 = Absolute Value(x=w952) -> (abs(x)=w948:dbl[])
                      n583 = Add Array Elements(numeric array=w948) -> (sum=w947:dbl)
                      n584 = Add Array Elements(numeric array=w950) -> (sum=w941:dbl)
                      n585 = Add Array Elements(numeric array=w949) -> (sum=w943:dbl)
                      n586 = Divide(x=w947, y=3.0) -> (x/y=w935:dbl)
                      n587 = Round To Nearest(number=w941) -> (nearest integer value=w940:dbl)
                      n588 = Round To Nearest(number=w943) -> (nearest integer value=w942:dbl)
                      n589 = Multiply(x=w935, y=w934) -> (x*y=w936:dbl)
                      n590 = Round To Nearest(number=w936) -> (nearest integer value=w937:dbl)
                      n591 = Divide(x=w940, y=w934) -> (x/y=→"kW":dbl)
                      n592 = Divide(x=w942, y=w934) -> (x/y=→"?VkVAr":dbl)
                      n593 = Divide(x=w937, y=w934) -> (x/y=w938:dbl)
                      n594 = node(w938) -> (→"A":dbl[unit])
                    }
                    frame 16 {
                      w953 = 1000.0 ("y")
                      n595 = Complex To Re/Im(x + iy=w970) -> (x=w969:dbl[], y=w968:dbl[])
                      n596 = Absolute Value(x=w971) -> (abs(x)=w967:dbl[])
                      n597 = Add Array Elements(numeric array=w967) -> (sum=w966:dbl)
                      n598 = Add Array Elements(numeric array=w969) -> (sum=w960:dbl)
                      n599 = Add Array Elements(numeric array=w968) -> (sum=w962:dbl)
                      n600 = Divide(x=w966, y=3.0) -> (x/y=w954:dbl)
                      n601 = Round To Nearest(number=w960) -> (nearest integer value=w959:dbl)
                      n602 = Round To Nearest(number=w962) -> (nearest integer value=w961:dbl)
                      n603 = Multiply(x=w954, y=w953) -> (x*y=w955:dbl)
                      n604 = Round To Nearest(number=w955) -> (nearest integer value=w956:dbl)
                      n605 = Divide(x=w959, y=w953) -> (x/y=→"kW":dbl)
                      n606 = Divide(x=w961, y=w953) -> (x/y=→"?VkVAr":dbl)
                      n607 = Divide(x=w956, y=w953) -> (x/y=w957:dbl)
                      n608 = node(w957) -> (→"A":dbl[unit])
                    }
                    frame 17 {
                      w972 = 1000.0 ("y")
                      n609 = Complex To Re/Im(x + iy=w989) -> (x=w988:dbl[], y=w987:dbl[])
                      n610 = Absolute Value(x=w990) -> (abs(x)=w986:dbl[])
                      n611 = Add Array Elements(numeric array=w986) -> (sum=w985:dbl)
                      n612 = Add Array Elements(numeric array=w988) -> (sum=w979:dbl)
                      n613 = Add Array Elements(numeric array=w987) -> (sum=w981:dbl)
                      n614 = Divide(x=w985, y=3.0) -> (x/y=w973:dbl)
                      n615 = Round To Nearest(number=w979) -> (nearest integer value=w978:dbl)
                      n616 = Round To Nearest(number=w981) -> (nearest integer value=w980:dbl)
                      n617 = Multiply(x=w973, y=w972) -> (x*y=w974:dbl)
                      n618 = Round To Nearest(number=w974) -> (nearest integer value=w975:dbl)
                      n619 = Divide(x=w978, y=w972) -> (x/y=→"kW":dbl)
                      n620 = Divide(x=w980, y=w972) -> (x/y=→"?VkVAr":dbl)
                      n621 = Divide(x=w975, y=w972) -> (x/y=w976:dbl)
                      n622 = node(w976) -> (→"A":dbl[unit])
                    }
                    frame 18 {
                      w998 = 1000.0 ("y")
                      n623 = Index Array(array=w993) -> (element=w992:cdb)  [unwired: 1 in]
                      n624 = Index Array(array=w995) -> (element=w994:cdb)  [unwired: 1 in]
                      n625 = Absolute Value(x=w992) -> (abs(x)=w997:dbl)
                      n626 = Absolute Value(x=w994) -> (abs(x)=w996:dbl)
                      n627 = Round To Nearest(number=w996) -> (nearest integer value=w1002:dbl)
                      n628 = Multiply(x=w997, y=w998) -> (x*y=w999:dbl)
                      n629 = Round To Nearest(number=w999) -> (nearest integer value=w1000:dbl)
                      n630 = Divide(x=w1002, y=w998) -> (x/y=→"kW":dbl)
                      n631 = Divide(x=w1000, y=w998) -> (x/y=→"A":dbl)
                    }
                    frame 19 {
                      w1010 = 1000.0 ("y")
                      n632 = Index Array(array=w1005) -> (element=w1004:cdb)  [unwired: 1 in]
                      n633 = Index Array(array=w1007) -> (element=w1006:cdb)  [unwired: 1 in]
                      n634 = Absolute Value(x=w1004) -> (abs(x)=w1009:dbl)
                      n635 = Absolute Value(x=w1006) -> (abs(x)=w1008:dbl)
                      n636 = Round To Nearest(number=w1008) -> (nearest integer value=w1014:dbl)
                      n637 = Multiply(x=w1009, y=w1010) -> (x*y=w1011:dbl)
                      n638 = Round To Nearest(number=w1011) -> (nearest integer value=w1012:dbl)
                      n639 = Divide(x=w1014, y=w1010) -> (x/y=→"kW":dbl)
                      n640 = Divide(x=w1012, y=w1010) -> (x/y=→"A":dbl)
                    }
                    frame 20 {
                      w1022 = 1000.0 ("y")
                      n641 = Index Array(array=w1017) -> (element=w1016:cdb)  [unwired: 1 in]
                      n642 = Index Array(array=w1019) -> (element=w1018:cdb)  [unwired: 1 in]
                      n643 = Absolute Value(x=w1016) -> (abs(x)=w1021:dbl)
                      n644 = Absolute Value(x=w1018) -> (abs(x)=w1020:dbl)
                      n645 = Round To Nearest(number=w1020) -> (nearest integer value=w1026:dbl)
                      n646 = Multiply(x=w1021, y=w1022) -> (x*y=w1023:dbl)
                      n647 = Round To Nearest(number=w1023) -> (nearest integer value=w1024:dbl)
                      n648 = Divide(x=w1026, y=w1022) -> (x/y=→"kW":dbl)
                      n649 = Divide(x=w1024, y=w1022) -> (x/y=→"A":dbl)
                    }
                    frame 21 {
                      w1034 = 1000.0 ("y")
                      n650 = Index Array(array=w1029) -> (element=w1028:cdb)  [unwired: 1 in]
                      n651 = Index Array(array=w1031) -> (element=w1030:cdb)  [unwired: 1 in]
                      n652 = Absolute Value(x=w1028) -> (abs(x)=w1033:dbl)
                      n653 = Absolute Value(x=w1030) -> (abs(x)=w1032:dbl)
                      n654 = Round To Nearest(number=w1032) -> (nearest integer value=w1038:dbl)
                      n655 = Multiply(x=w1033, y=w1034) -> (x*y=w1035:dbl)
                      n656 = Round To Nearest(number=w1035) -> (nearest integer value=w1036:dbl)
                      n657 = Divide(x=w1038, y=w1034) -> (x/y=→"kW":dbl)
                      n658 = Divide(x=w1036, y=w1034) -> (x/y=→"A":dbl)
                    }
                    frame 22 {
                      w1046 = 1000.0 ("y")
                      n659 = Index Array(array=w1041) -> (element=w1040:cdb)  [unwired: 1 in]
                      n660 = Index Array(array=w1043) -> (element=w1042:cdb)  [unwired: 1 in]
                      n661 = Absolute Value(x=w1040) -> (abs(x)=w1045:dbl)
                      n662 = Absolute Value(x=w1042) -> (abs(x)=w1044:dbl)
                      n663 = Round To Nearest(number=w1044) -> (nearest integer value=w1050:dbl)
                      n664 = Multiply(x=w1045, y=w1046) -> (x*y=w1047:dbl)
                      n665 = Round To Nearest(number=w1047) -> (nearest integer value=w1048:dbl)
                      n666 = Divide(x=w1050, y=w1046) -> (x/y=→"kW":dbl)
                      n667 = Divide(x=w1048, y=w1046) -> (x/y=→"A":dbl)
                    }
                    frame 23 {
                      w1058 = 1000.0 ("y")
                      n668 = Index Array(array=w1053) -> (element=w1052:cdb)  [unwired: 1 in]
                      n669 = Index Array(array=w1055) -> (element=w1054:cdb)  [unwired: 1 in]
                      n670 = Absolute Value(x=w1052) -> (abs(x)=w1057:dbl)
                      n671 = Absolute Value(x=w1054) -> (abs(x)=w1056:dbl)
                      n672 = Round To Nearest(number=w1056) -> (nearest integer value=w1062:dbl)
                      n673 = Multiply(x=w1057, y=w1058) -> (x*y=w1059:dbl)
                      n674 = Round To Nearest(number=w1059) -> (nearest integer value=w1060:dbl)
                      n675 = Divide(x=w1062, y=w1058) -> (x/y=→"kW":dbl)
                      n676 = Divide(x=w1060, y=w1058) -> (x/y=→"A":dbl)
                    }
                    frame 24 {
                      w1070 = 1000.0 ("y")
                      n677 = Index Array(array=w1065) -> (element=w1064:cdb)  [unwired: 1 in]
                      n678 = Index Array(array=w1067) -> (element=w1066:cdb)  [unwired: 1 in]
                      n679 = Absolute Value(x=w1064) -> (abs(x)=w1069:dbl)
                      n680 = Absolute Value(x=w1066) -> (abs(x)=w1068:dbl)
                      n681 = Round To Nearest(number=w1068) -> (nearest integer value=w1074:dbl)
                      n682 = Multiply(x=w1069, y=w1070) -> (x*y=w1071:dbl)
                      n683 = Round To Nearest(number=w1071) -> (nearest integer value=w1072:dbl)
                      n684 = Divide(x=w1074, y=w1070) -> (x/y=→"kW":dbl)
                      n685 = Divide(x=w1072, y=w1070) -> (x/y=→"A":dbl)
                    }
                    frame 25 {
                      w1082 = 1000.0 ("y")
                      n686 = Index Array(array=w1077) -> (element=w1076:cdb)  [unwired: 1 in]
                      n687 = Index Array(array=w1079) -> (element=w1078:cdb)  [unwired: 1 in]
                      n688 = Absolute Value(x=w1076) -> (abs(x)=w1081:dbl)
                      n689 = Absolute Value(x=w1078) -> (abs(x)=w1080:dbl)
                      n690 = Round To Nearest(number=w1080) -> (nearest integer value=w1086:dbl)
                      n691 = Multiply(x=w1081, y=w1082) -> (x*y=w1083:dbl)
                      n692 = Round To Nearest(number=w1083) -> (nearest integer value=w1084:dbl)
                      n693 = Divide(x=w1086, y=w1082) -> (x/y=→"kW":dbl)
                      n694 = Divide(x=w1084, y=w1082) -> (x/y=→"A":dbl)
                    }
                  }
                }
              }
            }
            n695 = for {
              tunnel: w454 -> [w463] mode=indexing
              i -> [w462]
              n696 = Unbundle By Name(w463) -> ("Vbus"=w461:cdb[], "Vband"=w458:T4)
              n697 = call "Plot Nodal Voltage.vi"("Range"=w458, "Voltage"=w461) -> ("Vp"=w459:dbl, "Vm"=w460:T8)
              n698 = case shown="True" TRUE {
                tunnel: w460 -> [_ w466]
                tunnel: w462 -> [_ w465]
                tunnel: w459 -> [_ w464]
                frame False {
                }
                frame True {
                  n699 = case shown="4" w465 {
                    tunnel: w466 -> [w474 w482 w490 w498 w506 _ w514 w522 w530 w538 w546 w564 w572 w580 w588 w596 w604 w612 w619 w626 w633 w640 w647 w654 w661 w668 _]
                    tunnel: w464 -> [_ _ _ _ _ _ _ _ _ _ _ _ _ _ _ _ _ _ _ _ _ _ _ _ _ _ _]
                    frame 0 {
                      n700 = Unbundle By Name(w474) -> ("Phasor C"=w473:dbl, "Phasor C"=w468:dbl, "Phasor C"=w467:dbl)
                      n701 = Absolute Value(x=w473) -> (abs(x)=w471:dbl)
                      n702 = Absolute Value(x=w468) -> (abs(x)=w470:dbl)
                      n703 = Absolute Value(x=w467) -> (abs(x)=w469:dbl)
                      n704 = Bundle(w471, w470, w469) -> (→"V slider 0":cluster{dbl, dbl, dbl})  [unwired: 1 in]
                    }
                    frame 1 {
                      n705 = Unbundle By Name(w482) -> ("Phasor C"=w481:dbl, "Phasor C"=w476:dbl, "Phasor C"=w475:dbl)
                      n706 = Absolute Value(x=w481) -> (abs(x)=w479:dbl)
                      n707 = Absolute Value(x=w476) -> (abs(x)=w478:dbl)
                      n708 = Absolute Value(x=w475) -> (abs(x)=w477:dbl)
                      n709 = Bundle(w479, w478, w477) -> (→"V slider 1":cluster{dbl, dbl, dbl})  [unwired: 1 in]
                    }
                    frame 2 {
                      n710 = Unbundle By Name(w490) -> ("Phasor C"=w489:dbl, "Phasor C"=w484:dbl, "Phasor C"=w483:dbl)
                      n711 = Absolute Value(x=w489) -> (abs(x)=w487:dbl)
                      n712 = Absolute Value(x=w484) -> (abs(x)=w486:dbl)
                      n713 = Absolute Value(x=w483) -> (abs(x)=w485:dbl)
                      n714 = Bundle(w487, w486, w485) -> (→"V slider 2":cluster{dbl, dbl, dbl})  [unwired: 1 in]
                    }
                    frame 3 {
                      n715 = Unbundle By Name(w498) -> ("Phasor C"=w497:dbl, "Phasor C"=w492:dbl, "Phasor C"=w491:dbl)
                      n716 = Absolute Value(x=w497) -> (abs(x)=w495:dbl)
                      n717 = Absolute Value(x=w492) -> (abs(x)=w494:dbl)
                      n718 = Absolute Value(x=w491) -> (abs(x)=w493:dbl)
                      n719 = Bundle(w495, w494, w493) -> (→"V slider 3":cluster{dbl, dbl, dbl})  [unwired: 1 in]
                    }
                    frame 4 {
                      n720 = Unbundle By Name(w506) -> ("Phasor C"=w505:dbl, "Phasor C"=w500:dbl, "Phasor C"=w499:dbl)
                      n721 = Absolute Value(x=w505) -> (abs(x)=w503:dbl)
                      n722 = Absolute Value(x=w500) -> (abs(x)=w502:dbl)
                      n723 = Absolute Value(x=w499) -> (abs(x)=w501:dbl)
                      n724 = Bundle(w503, w502, w501) -> (→"V slider 4":cluster{dbl, dbl, dbl})  [unwired: 1 in]
                    }
                    frame 5 {
                    }
                    frame 6 {
                      n725 = Unbundle By Name(w514) -> ("Phasor C"=w513:dbl, "Phasor C"=w508:dbl, "Phasor C"=w507:dbl)
                      n726 = Absolute Value(x=w513) -> (abs(x)=w511:dbl)
                      n727 = Absolute Value(x=w508) -> (abs(x)=w510:dbl)
                      n728 = Absolute Value(x=w507) -> (abs(x)=w509:dbl)
                      n729 = Bundle(w511, w510, w509) -> (→"V slider 6":cluster{dbl, dbl, dbl})  [unwired: 1 in]
                    }
                    frame 7 {
                      n730 = Unbundle By Name(w522) -> ("Phasor C"=w521:dbl, "Phasor C"=w516:dbl, "Phasor C"=w515:dbl)
                      n731 = Absolute Value(x=w521) -> (abs(x)=w519:dbl)
                      n732 = Absolute Value(x=w516) -> (abs(x)=w518:dbl)
                      n733 = Absolute Value(x=w515) -> (abs(x)=w517:dbl)
                      n734 = Bundle(w519, w518, w517) -> (→"V slider 7":cluster{dbl, dbl, dbl})  [unwired: 1 in]
                    }
                    frame 8 {
                      n735 = Unbundle By Name(w530) -> ("Phasor C"=w529:dbl, "Phasor C"=w524:dbl, "Phasor C"=w523:dbl)
                      n736 = Absolute Value(x=w529) -> (abs(x)=w527:dbl)
                      n737 = Absolute Value(x=w524) -> (abs(x)=w526:dbl)
                      n738 = Absolute Value(x=w523) -> (abs(x)=w525:dbl)
                      n739 = Bundle(w527, w526, w525) -> (→"V slider 8":cluster{dbl, dbl, dbl})  [unwired: 1 in]
                    }
                    frame 9 {
                      n740 = Unbundle By Name(w538) -> ("Phasor C"=w537:dbl, "Phasor C"=w532:dbl, "Phasor C"=w531:dbl)
                      n741 = Absolute Value(x=w537) -> (abs(x)=w535:dbl)
                      n742 = Absolute Value(x=w532) -> (abs(x)=w534:dbl)
                      n743 = Absolute Value(x=w531) -> (abs(x)=w533:dbl)
                      n744 = Bundle(w535, w534, w533) -> (→"V slider 9":cluster{dbl, dbl, dbl})  [unwired: 1 in]
                    }
                    frame 10 {
                      n745 = Unbundle By Name(w546) -> ("Phasor C"=w545:dbl, "Phasor C"=w540:dbl, "Phasor C"=w539:dbl)
                      n746 = Absolute Value(x=w545) -> (abs(x)=w543:dbl)
                      n747 = Absolute Value(x=w540) -> (abs(x)=w542:dbl)
                      n748 = Absolute Value(x=w539) -> (abs(x)=w541:dbl)
                      n749 = Bundle(w543, w542, w541) -> (→"V slider 10":cluster{dbl, dbl, dbl})  [unwired: 1 in]
                    }
                    frame 11 {
                      w547 = 10.0 ("y")
                      n750 = Unbundle By Name(w564) -> ("Phasor C"=w563:dbl, "Phasor C"=w561:dbl, "Phasor C"=w560:dbl)
                      n751 = Absolute Value(x=w563) -> (abs(x)=w559:dbl)
                      n752 = Absolute Value(x=w561) -> (abs(x)=w551:dbl)
                      n753 = Absolute Value(x=w560) -> (abs(x)=w550:dbl)
                      n754 = Multiply(x=w559, y=w547) -> (x*y=w558:dbl)
                      n755 = Multiply(x=w551, y=w547) -> (x*y=w555:dbl)
                      n756 = Multiply(x=w550, y=w547) -> (x*y=w553:dbl)
                      n757 = Round To Nearest(number=w558) -> (nearest integer value=w557:dbl)
                      n758 = Round To Nearest(number=w555) -> (nearest integer value=w554:dbl)
                      n759 = Round To Nearest(number=w553) -> (nearest integer value=w552:dbl)
                      n760 = Divide(x=w557, y=w547) -> (x/y=w556:dbl)
                      n761 = Divide(x=w554, y=w547) -> (x/y=w549:dbl)
                      n762 = Divide(x=w552, y=w547) -> (x/y=w548:dbl)
                      n763 = Bundle(w556, w549, w548) -> (→"V slider 11":cluster{dbl, dbl, dbl})  [unwired: 1 in]
                    }
                    frame 12 {
                      n764 = Unbundle By Name(w572) -> ("Phasor C"=w571:dbl, "Phasor C"=w566:dbl, "Phasor C"=w565:dbl)
                      n765 = Absolute Value(x=w571) -> (abs(x)=w569:dbl)
                      n766 = Absolute Value(x=w566) -> (abs(x)=w568:dbl)
                      n767 = Absolute Value(x=w565) -> (abs(x)=w567:dbl)
                      n768 = Bundle(w569, w568, w567) -> (→"V slider 12":cluster{dbl, dbl, dbl})  [unwired: 1 in]
                    }
                    frame 13 {
                      n769 = Unbundle By Name(w580) -> ("Phasor C"=w579:dbl, "Phasor C"=w574:dbl, "Phasor C"=w573:dbl)
                      n770 = Absolute Value(x=w579) -> (abs(x)=w577:dbl)
                      n771 = Absolute Value(x=w574) -> (abs(x)=w576:dbl)
                      n772 = Absolute Value(x=w573) -> (abs(x)=w575:dbl)
                      n773 = Bundle(w577, w576, w575) -> (→"V slider 13":cluster{dbl, dbl, dbl})  [unwired: 1 in]
                    }
                    frame 14 {
                      n774 = Unbundle By Name(w588) -> ("Phasor C"=w587:dbl, "Phasor C"=w582:dbl, "Phasor C"=w581:dbl)
                      n775 = Absolute Value(x=w587) -> (abs(x)=w585:dbl)
                      n776 = Absolute Value(x=w582) -> (abs(x)=w584:dbl)
                      n777 = Absolute Value(x=w581) -> (abs(x)=w583:dbl)
                      n778 = Bundle(w585, w584, w583) -> (→"V slider 14":cluster{dbl, dbl, dbl})  [unwired: 1 in]
                    }
                    frame 15 {
                      n779 = Unbundle By Name(w596) -> ("Phasor C"=w595:dbl, "Phasor C"=w590:dbl, "Phasor C"=w589:dbl)
                      n780 = Absolute Value(x=w595) -> (abs(x)=w593:dbl)
                      n781 = Absolute Value(x=w590) -> (abs(x)=w592:dbl)
                      n782 = Absolute Value(x=w589) -> (abs(x)=w591:dbl)
                      n783 = Bundle(w593, w592, w591) -> (→"V slider 15":cluster{dbl, dbl, dbl})  [unwired: 1 in]
                    }
                    frame 16 {
                      n784 = Unbundle By Name(w604) -> ("Phasor C"=w603:dbl, "Phasor C"=w598:dbl, "Phasor C"=w597:dbl)
                      n785 = Absolute Value(x=w603) -> (abs(x)=w601:dbl)
                      n786 = Absolute Value(x=w598) -> (abs(x)=w600:dbl)
                      n787 = Absolute Value(x=w597) -> (abs(x)=w599:dbl)
                      n788 = Bundle(w601, w600, w599) -> (→"V slider 16":cluster{dbl, dbl, dbl})  [unwired: 1 in]
                    }
                    frame 17 {
                      n789 = Unbundle By Name(w612) -> ("Phasor C"=w611:dbl, "Phasor C"=w606:dbl, "Phasor C"=w605:dbl)
                      n790 = Absolute Value(x=w611) -> (abs(x)=w609:dbl)
                      n791 = Absolute Value(x=w606) -> (abs(x)=w608:dbl)
                      n792 = Absolute Value(x=w605) -> (abs(x)=w607:dbl)
                      n793 = Bundle(w609, w608, w607) -> (→"V slider 17":cluster{dbl, dbl, dbl})  [unwired: 1 in]
                    }
                    frame 18 {
                      w615 = 10.0 ("y")
                      n794 = Unbundle By Name(w619) -> ("Phasor C"=w618:dbl)
                      n795 = Absolute Value(x=w618) -> (abs(x)=w614:dbl)
                      n796 = Multiply(x=w614, y=w615) -> (x*y=w617:dbl)
                      n797 = Round To Nearest(number=w617) -> (nearest integer value=w616:dbl)
                      n798 = Divide(x=w616, y=w615) -> (x/y=→"V slider 18":dbl)
                    }
                    frame 19 {
                      w622 = 10.0 ("y")
                      n799 = Unbundle By Name(w626) -> ("Phasor C"=w625:dbl)
                      n800 = Absolute Value(x=w625) -> (abs(x)=w621:dbl)
                      n801 = Multiply(x=w621, y=w622) -> (x*y=w624:dbl)
                      n802 = Round To Nearest(number=w624) -> (nearest integer value=w623:dbl)
                      n803 = Divide(x=w623, y=w622) -> (x/y=→"V slider 19":dbl)
                    }
                    frame 20 {
                      w629 = 10.0 ("y")
                      n804 = Unbundle By Name(w633) -> ("Phasor C"=w632:dbl)
                      n805 = Absolute Value(x=w632) -> (abs(x)=w628:dbl)
                      n806 = Multiply(x=w628, y=w629) -> (x*y=w631:dbl)
                      n807 = Round To Nearest(number=w631) -> (nearest integer value=w630:dbl)
                      n808 = Divide(x=w630, y=w629) -> (x/y=→"V slider 20":dbl)
                    }
                    frame 21 {
                      w636 = 10.0 ("y")
                      n809 = Unbundle By Name(w640) -> ("Phasor C"=w639:dbl)
                      n810 = Absolute Value(x=w639) -> (abs(x)=w635:dbl)
                      n811 = Multiply(x=w635, y=w636) -> (x*y=w638:dbl)
                      n812 = Round To Nearest(number=w638) -> (nearest integer value=w637:dbl)
                      n813 = Divide(x=w637, y=w636) -> (x/y=→"V slider 21":dbl)
                    }
                    frame 22 {
                      w643 = 10.0 ("y")
                      n814 = Unbundle By Name(w647) -> ("Phasor C"=w646:dbl)
                      n815 = Absolute Value(x=w646) -> (abs(x)=w642:dbl)
                      n816 = Multiply(x=w642, y=w643) -> (x*y=w645:dbl)
                      n817 = Round To Nearest(number=w645) -> (nearest integer value=w644:dbl)
                      n818 = Divide(x=w644, y=w643) -> (x/y=→"V slider 22":dbl)
                    }
                    frame 23 {
                      w650 = 10.0 ("y")
                      n819 = Unbundle By Name(w654) -> ("Phasor C"=w653:dbl)
                      n820 = Absolute Value(x=w653) -> (abs(x)=w649:dbl)
                      n821 = Multiply(x=w649, y=w650) -> (x*y=w652:dbl)
                      n822 = Round To Nearest(number=w652) -> (nearest integer value=w651:dbl)
                      n823 = Divide(x=w651, y=w650) -> (x/y=→"V slider 23":dbl)
                    }
                    frame 24 {
                      w657 = 10.0 ("y")
                      n824 = Unbundle By Name(w661) -> ("Phasor C"=w660:dbl)
                      n825 = Absolute Value(x=w660) -> (abs(x)=w656:dbl)
                      n826 = Multiply(x=w656, y=w657) -> (x*y=w659:dbl)
                      n827 = Round To Nearest(number=w659) -> (nearest integer value=w658:dbl)
                      n828 = Divide(x=w658, y=w657) -> (x/y=→"V slider 24":dbl)
                    }
                    frame 25 {
                      w664 = 10.0 ("y")
                      n829 = Unbundle By Name(w668) -> ("Phasor C"=w667:dbl)
                      n830 = Absolute Value(x=w667) -> (abs(x)=w663:dbl)
                      n831 = Multiply(x=w663, y=w664) -> (x*y=w666:dbl)
                      n832 = Round To Nearest(number=w666) -> (nearest integer value=w665:dbl)
                      n833 = Divide(x=w665, y=w664) -> (x/y=→"V slider 25":dbl)
                    }
                    frame 26, Default {
                    }
                  }
                }
              }
            }
          }
          frame True {
          }
        }
        n834 = Wait on Notification(notifier=w448, timeout in ms (-1)=w442, error in (no error)=w446) -> (notifier out=w447:refnum<notifier>, notification=w441:bool, error out=w445:errorcluster)  [unwired: 1 in, 1 out]
        n835 = local write "Stop?"(w441) -> ()
        n836 = Wait (ms)(milliseconds to wait=u32 5) -> ()  [unwired: 1 out]
      }
      n837 = UDP Open(8:w419, 11:u16 54321 ("port")) -> (port=w422:refnum<k16>, 0:w420:errorcluster)  [unwired: 3 in, 1 out]
      n838 = while {
        shift-right: [w432] -> w421
        shift-left: w420 -> [w439]
        shift-right: [w436] -> w423
        shift-left: w422 -> [w438]
        stop <- "Stop?" stop-if-true
        # "Receive"
        n839 = UDP Read(connection ID=w438, timeout ms (25000)=-1, 8:w439) -> (data out=w435:string, error out=w433:errorcluster, 3:w436:refnum<k16>)  [unwired: 1 in, 2 out]
        n840 = Unflatten From JSON(JSON string=w435, type and defaults=cluster{"Connected?":bool} {"Connected?"=TRUE}, error in (no error)=w433) -> (value=w430:cluster{"Connected?":bool}, error out=w432:errorcluster)  [unwired: 4 in]
        n841 = Unbundle By Name(w430) -> ("Connected?"=→"Connected?":bool)
      }
      n842 = UDP Close(connection ID=w423, 8:w421) -> (error out=w416:errorcluster)  [unwired: 1 out]
      n843 = Merge Errors(w418, w416) -> (w417:errorcluster)
    }
  }
  "Stop (Out)" <- w9
  "Error (Out)" <- w4
  "SCADA AugState (Out)" <- w2
